vi "handleMode.vi"(8 "error in (no error)":errorcluster, 10 "stepName":T1, 11 "Stand in":refnum<class "Stand.lvclass">) -> (0 "error out":errorcluster, 3 "Stand out":refnum<class "Stand.lvclass">)   [LabVIEW 2019, in "Stand.lvclass"]
uses:
  Stand.lvclass
  FPGA/TypeDef/DO index.ctl
  Valve_2DO_2DI_class/Valve_2DO_2DI.lvclass
  TypeDef/Direction.ctl
  Device_class/Device.lvclass
  FPGA_API_class/FPGA API.lvclass
  f638fa31-f737-482a-bde8-81f5a2056bae.vi
  PM_Group_class/PM_Group.lvclass
  TypeDef/Motor N.ctl
  TypeDef/Active Motor.ctl
  MessageInterface_class/MessageInterface.lvclass
  TypeDef/Step_Name.ctl
  FPGA/TypeDef/AI index.ctl
  AI_class/AI.lvclass
  NeedleValve_class/NeedleValve.lvclass
  D:/GIT H4000/H4000/src/Device_class/Device.lvclass
  D:/GIT H4000/H4000/src/Proccess_class/Proccess.lvclass
  ExpFitter/ExpFitter.lvclass
  TypeDef/Needle Valve State.ctl
  LinealFitting/LinealFitting.lvclass
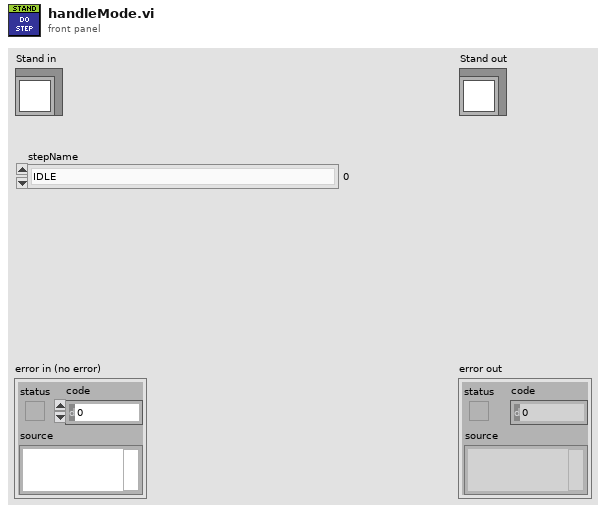
[diagram p1: front panel]
types:
  T1 = typedef "Step_Name.ctl" = enum16{"IDLE", "Filling", "Low Pressure", "Hi Pressure", "Abrupt Pressure Release", "Smooth Pressure Release", "Measuring Leakage Sensor 41.3", "Measuring Leakage Burette 42", "Alarm", "Stop Pump"}
  T2 = typedef "Direction.ctl" = enum16{"None", "DUT", "Chamber"}
  T3 = typedef "Active Motor.ctl" = cluster{"Active":bool, "MotorN":T4}
  T4 = typedef "Motor N.ctl" = enum16{"M12", "M21", "M24"}
  T5 = typedef "Step_Name.ctl" = enum16{"NONE", "Filling DUT", "Filling Chamber", "Pressure Up DUT", "Abrupt Pressure Release DUT", "Smooth Pressure Release DUT", "Pressure Up Chamber", "Abrupt Pressure Release Chamber", "Smooth Pressure Release Chamber", "Measuring leakage sensor 41.3", "Measuring leakage burette 42", "Low Pressure DUT", "Low Pressure Chamber", "Low Pressure HPP", "ALARM", "Open Air", "MicroStep DUT", "MicroStep CMBR", "Stop Pump", "Press Down by Valve DUT"}
  T6 = typedef "Needle Valve State.ctl" = enum16{"STOPED", "CLOSED", "OPENED", "OPENING", "CLOSING"}
  T7 = typedef "DO index.ctl" = u8
  T8 = typedef "AI index.ctl" = u8
  T9 = typedef "AI_Data.ctl" = cluster{"Stat Data":T10, "OutOfRangeMax":bool, "OutOfRangeMin":bool, "HIHI":bool, "HI":bool, "LO":bool, "LOLO":bool, "DATA N":T11, "DATA PERIOD":T11, "UPPER TH":dbl, "LOWER TH":dbl}
  T10 = typedef "AI Statistics Data.ctl" = cluster{"raw mean":dbl, "scl mean":dbl, "raw mean 1Hz":dbl, "scl mean 1Hz":dbl}
  T11 = typedef "DATA Oscill.ctl" = cluster{"SUM":dbl, "COUNTER":dbl, "MAX CURR":dbl, "MIN CURR":dbl, "AVR":dbl, "MAX":dbl, "MIN":dbl, "DELTA AVR":dbl, "DELTA MAX":dbl, "DELTA MIN":dbl, "PERIOD":dbl}
  T12 = typedef "Needle Valve Data.ctl" = cluster{"Engine State":T13, "StateValveModbus":T6, "Alarms":T14, "RAW":i32, "Angele":dbl, "Step":i32, "Encoder":i32, "Kinematic":T15, "Limits":T16, "EncoderMax":i32, "Counter Max Dont Update":i32, "EncoderMin":i32, "Counter Min Dont Update":i32, "Prepere Counter":i32, "STEP INIT":i32, "offset - Angel":dbl}
  T13 = typedef "MB_ENGINE.lvclass/Engine State.ctl" = u16
  T14 = typedef "MB_ENGINE.lvclass/Engine Alarms.ctl" = cluster{"OL":bool, "TF":bool, "STL":bool, "OCP":bool, "CPUV":bool, "UVLO":bool, "SPI_ERROR":bool, "Fault":bool, "OL 2":bool, "TF 2":bool, "STL 2":bool, "OCP 2":bool, "CPUV 2":bool, "UVLO 2":bool, "reserved":bool, "InitDone":bool}
  T15 = typedef "MB_ENGINE.lvclass/Settings.ctl" = cluster{"ACC Steps Per Sec^2":u16, "DEC Steps Per Sec^2":u16, "Min Velosity Step Per Sec":u16, "Max Velosity Step Per Sec":u16, "MicroStep":u16}
  T16 = typedef "MB_ENGINE.lvclass/Limits Status.ctl" = cluster{"Fault 2 Switch":bool, "Fault 1 Switch":bool, "Center(Home)":bool, "Lower Limit":bool, "Upper Limit":bool}
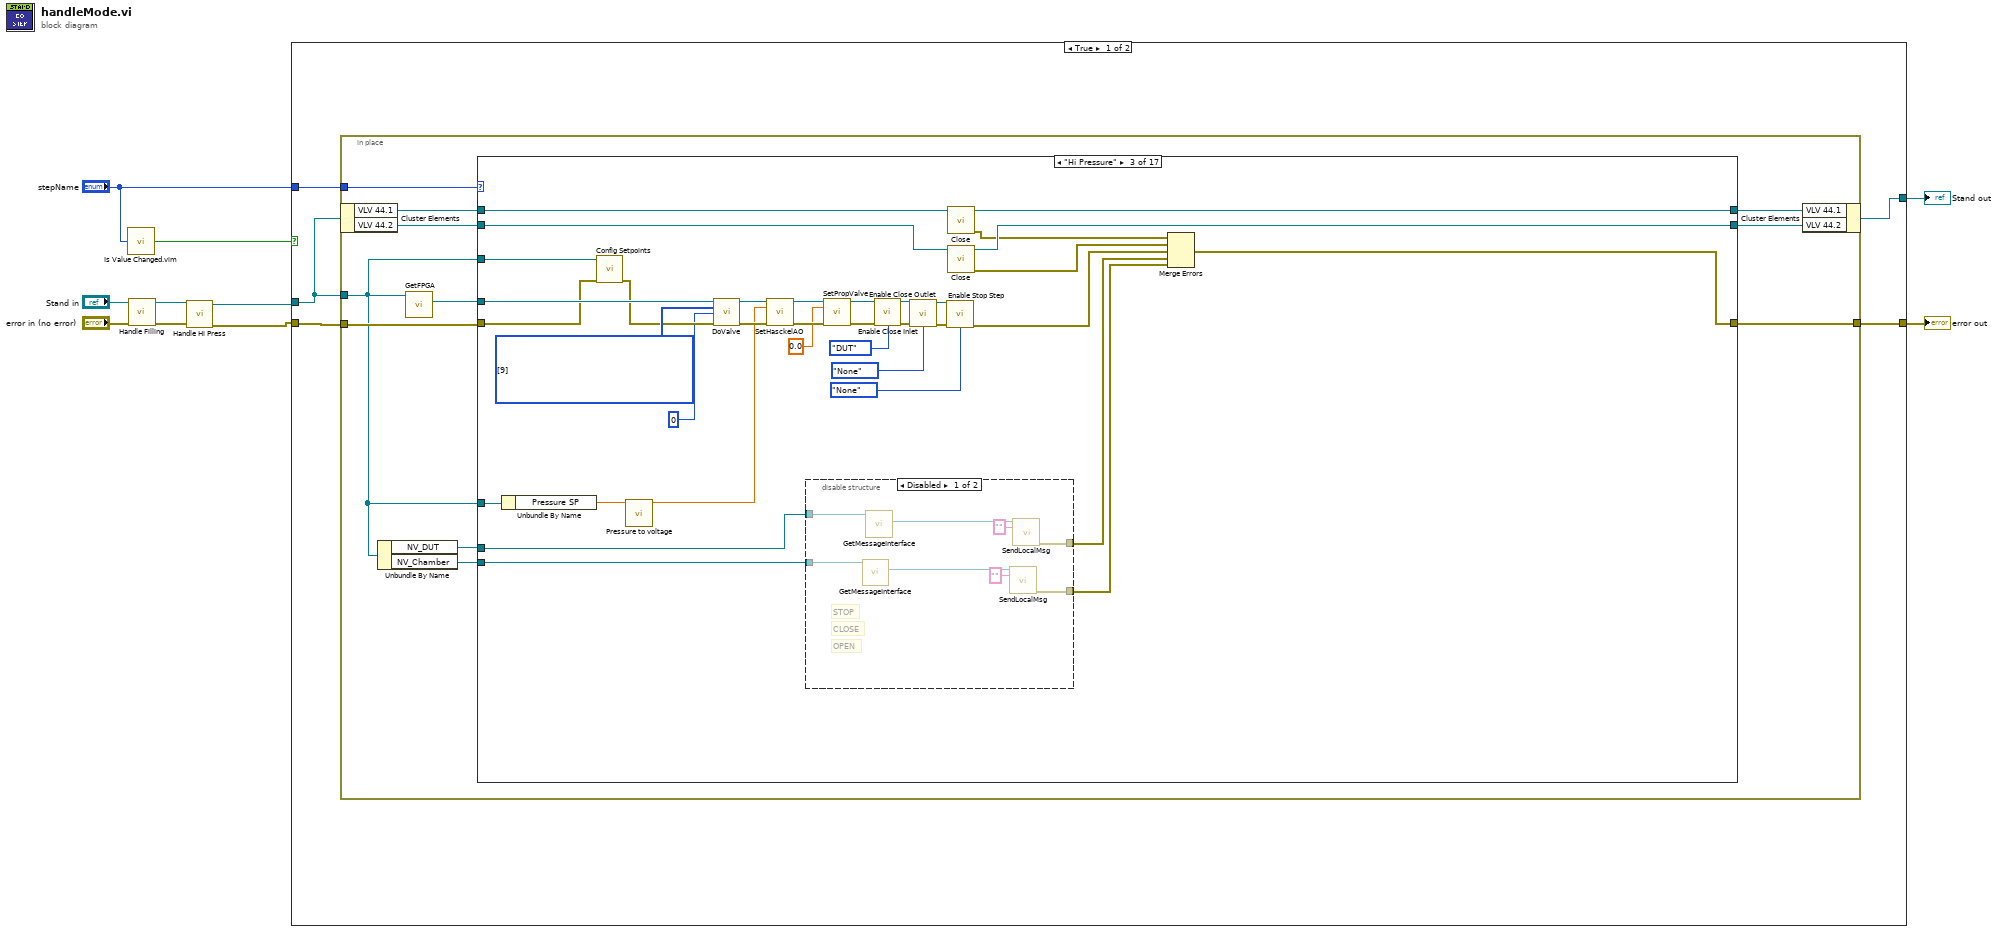
[diagram p0: block diagram]
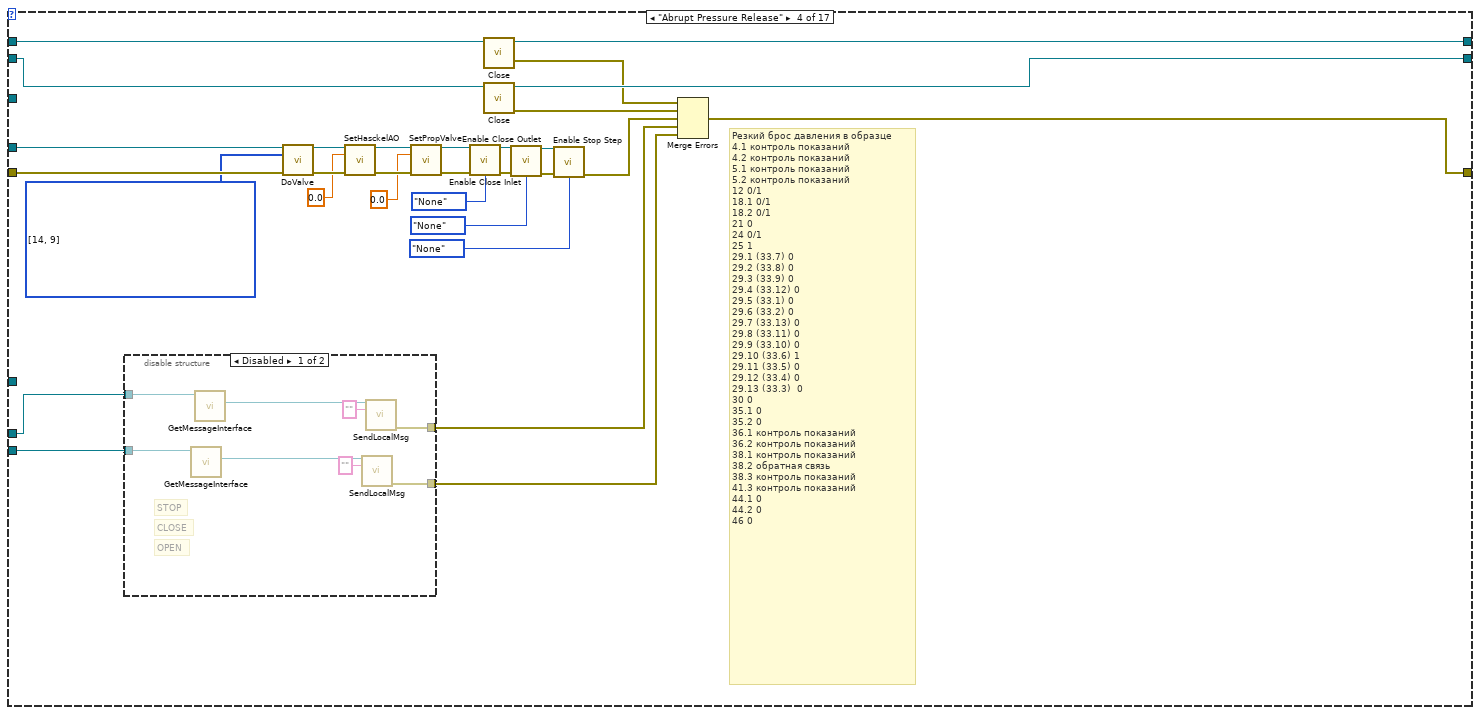
[diagram p5: hidden frame]
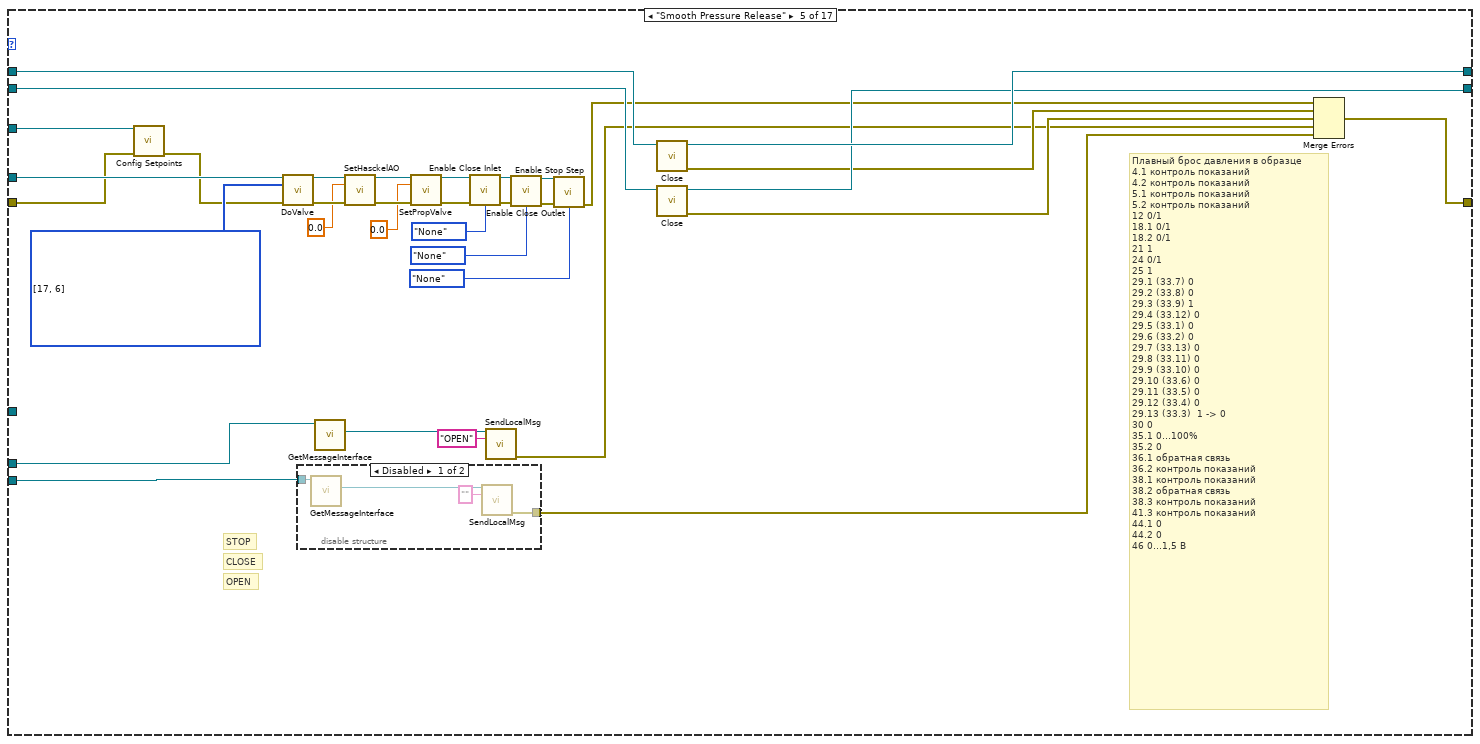
[diagram p7: hidden frame]
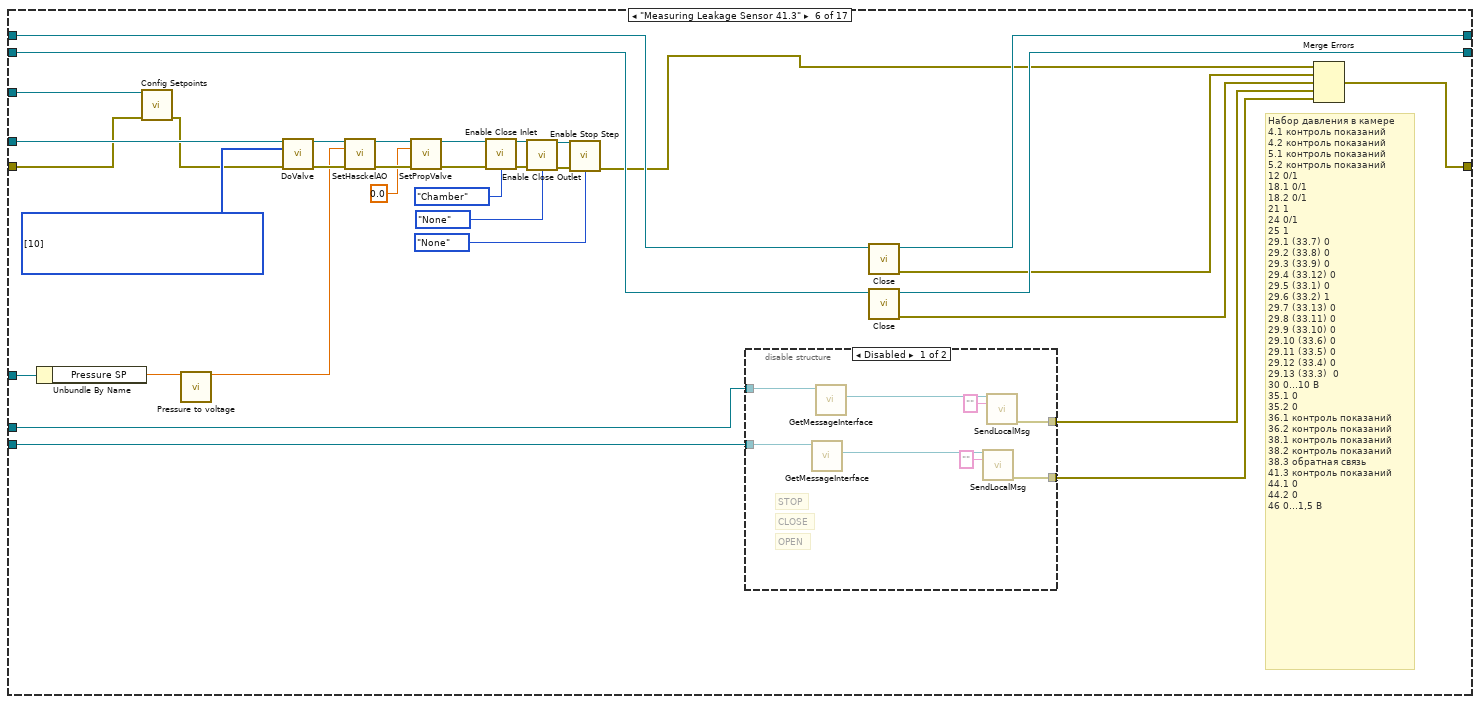
[diagram p9: hidden frame]
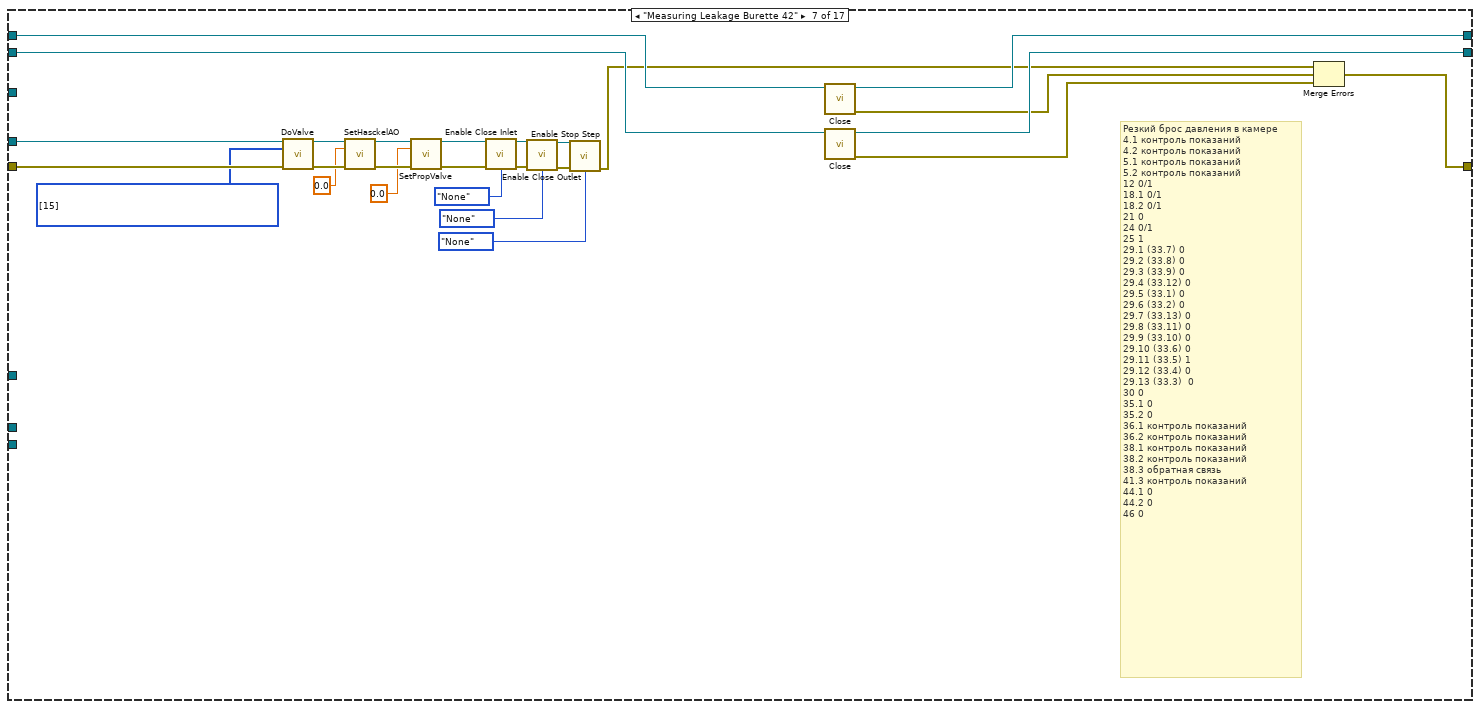
[diagram p11: hidden frame]
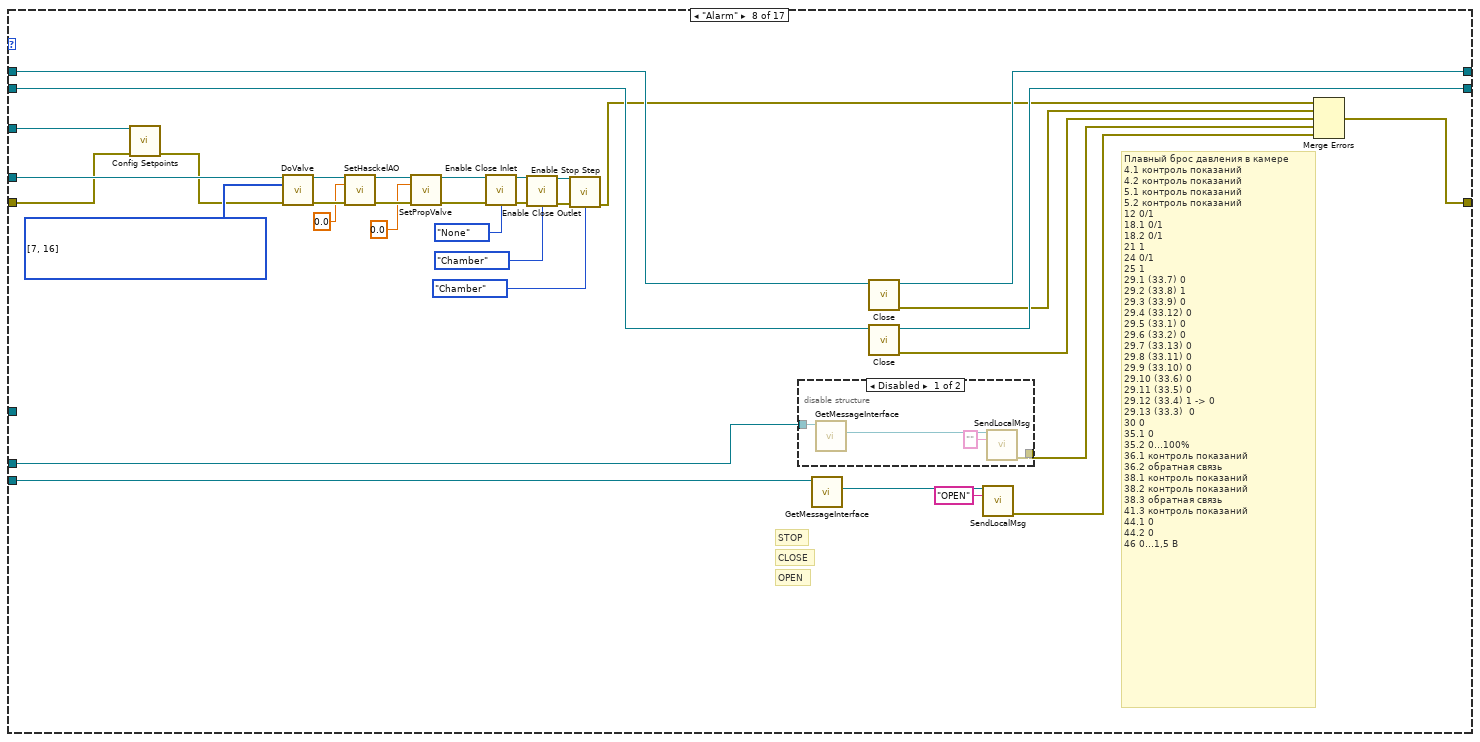
[diagram p12: hidden frame]
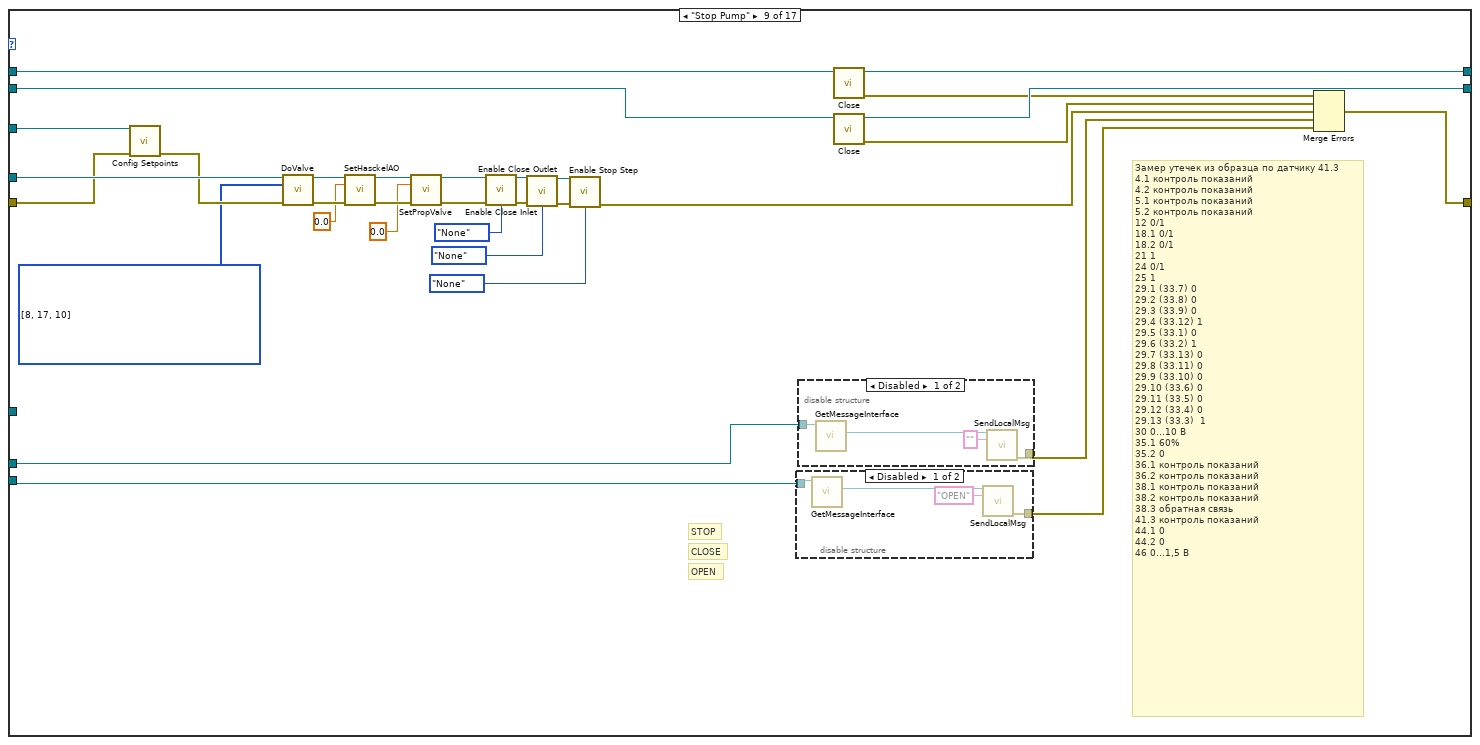
[diagram p14: hidden frame]
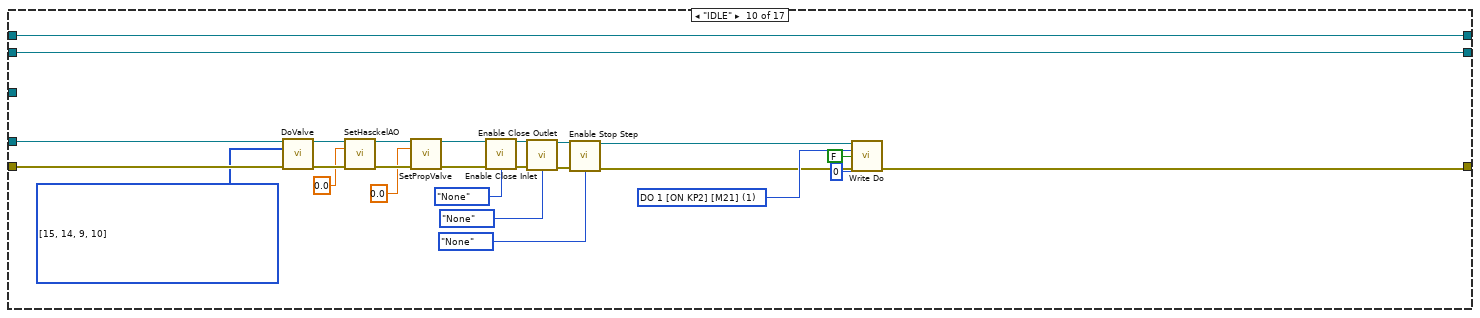
[diagram p17: hidden frame]
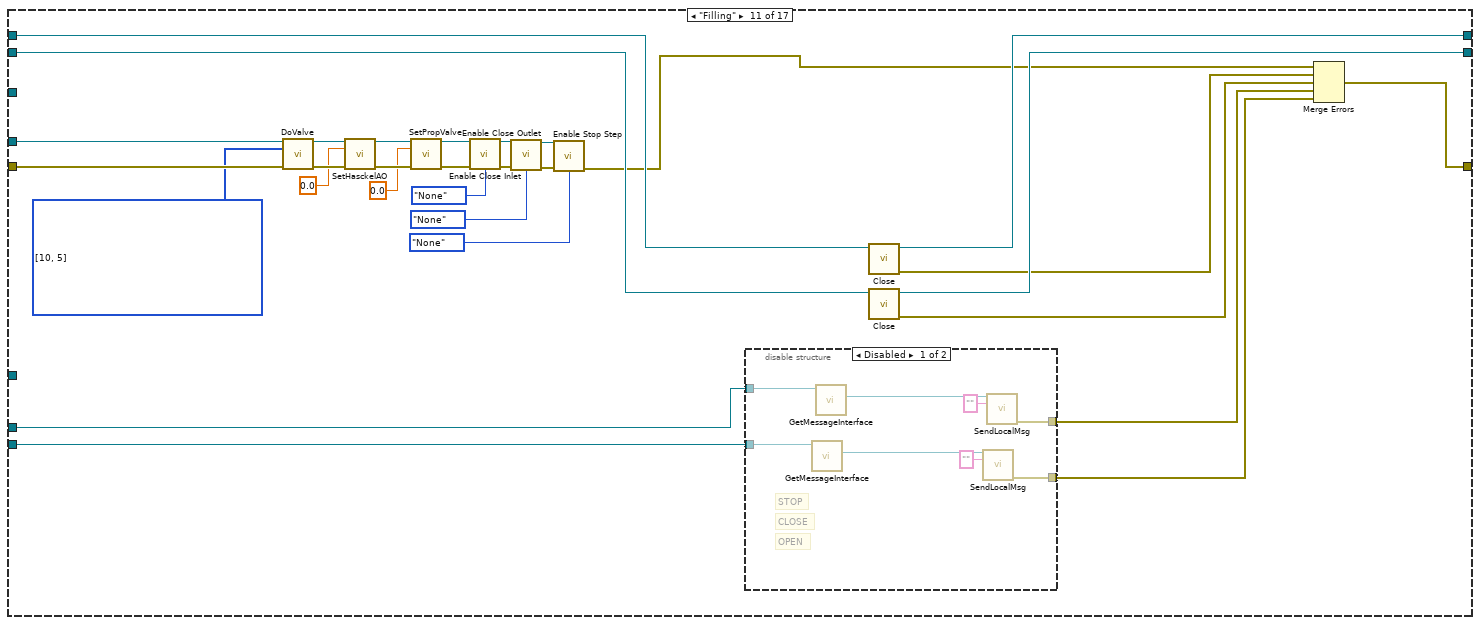
[diagram p18: hidden frame]
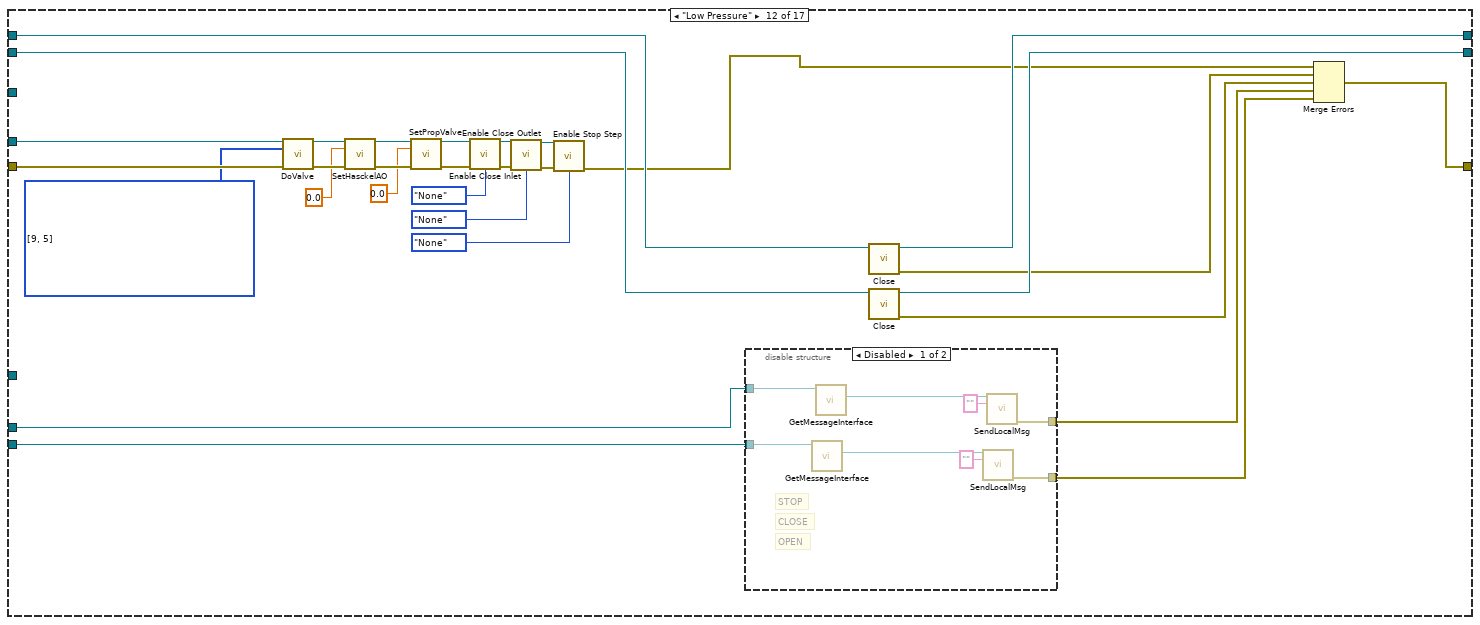
[diagram p20: hidden frame]
diagram:
  n1 = call "Is Value Changed.vim"("value"="stepName") -> ("changed or first call?"=w9:bool)
  n2 = call "Handle Filling.vi"("error in (no error)"="error in (no error)", "Stand in"="Stand in") -> ("error out"=w3:errorcluster, "Stand out"=w4:refnum<class "Stand.lvclass">)  [unwired: 8 in]
  n3 = call "Handle Hi Press.vi"("error in (no error)"=w3, "Stand in"=w4) -> ("error out"=w1:errorcluster, "Stand out"=w2:refnum<class "Stand.lvclass">)  [unwired: 8 in]
  n4 = case shown="True" w9 {
    tunnel: "stepName" -> [w15 _]
    tunnel: w2 -> [w13 w583]
    tunnel: w1 -> [w14 w584]
    tunnel: [w12 w582] -> w8
    tunnel: [w11 w581] -> w7
    frame True {
      n5 = in-place {
        in-place-border: w15 -> [w26]
        in-place-border: [w25] -> w11
        in-place-border: w14 -> [w24]
        in-place-border: w13 -> [w16]
        n6 = in-place-cluster #1(w13) -> ("VLV 44.1"=w22:refnum<class "Valve_2DO_2DI.lvclass">, "VLV 44.2"=w21:refnum<class "Valve_2DO_2DI.lvclass">)
        n7 = Unbundle By Name(w16) -> ("NV_DUT"=w18:refnum<class "NeedleValve.lvclass">, "NV_Chamber"=w17:refnum<class "NeedleValve.lvclass">)
        n8 = call "GetFPGA.vi"("Device in"=w16) -> ("FPGA API.lvclass"=w23:refnum<class "FPGA API.lvclass">)  [unwired: 10 in]
        n9 = case shown="\"Hi Pressure\"" w26 {
          tunnel: w24 -> [w29 _ w35 w102 w114 w150 w216 w218 w258 w320 w350 w388 w426 w437 w489 w523 w549]
          tunnel: [w29 _ w54 w92 w135 w172 w206 w241 w277 w296 w340 w378 w416 w458 w495 w529 w568] -> w25
          tunnel: w22 -> [w28 _ w59 w96 w139 w177 w210 w245 w281 w314 w344 w382 w420 w463 w505 w539 w570]
          tunnel: w21 -> [w27 _ w56 w94 w137 w174 w208 w243 w279 w313 w342 w380 w418 w460 w504 w538 w569]
          tunnel: w23 -> [_ _ w60 w97 w140 w178 w211 w246 w282 w315 w345 w383 w421 w464 w506 w540 w550]
          tunnel: w16 -> [_ _ w58 _ _ w176 _ _ _ _ _ _ _ w462 w482 w516 _]
          tunnel: [w28 _ w57 w95 w138 w175 w209 w244 w280 w314 w343 w381 w419 w461 w505 w539 w570] -> w20
          tunnel: [w27 _ w55 w93 w136 w173 w207 w242 w278 w313 w341 w379 w417 w459 w504 w538 w569] -> w19
          tunnel: w18 -> [_ _ w53 w91 w132 w169 _ w238 w274 _ w337 w375 w413 w455 _ _ w567]
          tunnel: w17 -> [_ _ w51 w89 w130 w167 _ w236 w272 _ w335 w373 w411 w453 _ _ w565]
          tunnel: w16 -> [_ _ w36 _ w115 w151 _ w219 w259 _ _ _ _ w438 w490 w524 _]
          frame "IDLE" {
          }
          frame "Low Pressure" {
          }
          frame "Hi Pressure" {
            w40 = T7[] [9] items=["DO 0 [KP1] [M12]", "DO 1 [ON KP2] [M21]", "DO 2 [ON KP3] [M24]", "DO 3 [WATER Y18.1 [DO3]]", "DO 4 [WATER Y18.2 [DO4]]", "DO 5 [KP6 Y29.1 33.7]", "DO 6 [KP7 Y29.2 33.8]", "DO 7 [KP8 Y29.3 33.9]", "DO 8 [KP9 Y29.4  33.12]", "DO 9 [KP10 Y29.5 33.1]", "DO 10 [KP11 Y29.6 33.2]", "DO 11 [KP12 Y29.7  33.13]", "DO 12 [KP13 Y29.8  33.11]", "DO 13 [KP14 Y29.9 33.10]", "DO 14 [KP15 Y29.10  33.6]", "DO 15 [KP16 Y29.11  33.5]", "DO 16 [KP17 Y29.12  33.4]", "DO 17 [KP18 Y29.13 33.3]", "DO 18 [AIR KP19]", "DO 19 [STEP DRIVE EN KP20]", "DO 20 [KP21 Y44.1 OPEN]", "DO 21 [ KP22 Y44.1 CLOSE]", "DO 22 [ KP23 Y44.2 OPEN]", "DO 23", "DO 24 [STEP DRIVE 1]", "DO 25 [STEP DRIVE 2]"] ("#DO")
            n10 = Unbundle By Name(w58) -> ("Pressure SP"=w38:dbl)
            n11 = call "Config Setpoints.vi"("reference in"=w36, "error in (no error)"=w35) -> ("error out"=w34:errorcluster)  [unwired: 13 in]
            n12 = call "Pressure to voltage.vi"("Pressure SP"=w38) -> ("Voltage"=w37:dbl)  [unwired: 14 in]
            n13 = call "DoValve.vi"("reference in"=w60, 5:w40, 7:u32 0 ("Time uSec"), "error in (no error)"=w34) -> ("reference out"=w64:refnum<class "FPGA API.lvclass">, "error out"=w63:errorcluster)  [unwired: 10 in]
            n14 = call-dynamic "SetHasckelAO.vi"("FPGA API in"=w64, "Haskel in"=w37, "error in (no error)"=w63) -> ("FPGA API out"=w62:refnum<class "FPGA API.lvclass">, "error out"=w61:errorcluster)  [unwired: 11 in]
            n15 = disable-structure shown="Disabled" {
              disable-tunnel: w53 -> [w72 _]
              disable-tunnel: [w70 _] -> w52
              disable-tunnel: w51 -> [w68 _]
              disable-tunnel: [w65 _] -> w41
              frame Disabled {
                # "OPEN"
                # "CLOSE"
                # "STOP"
                n16 = call "GetMessageInterface.vi"("Device in"=w68) -> ("MessageInterface"=w69:refnum<class "MessageInterface.lvclass">)  [unwired: 10 in]
                n17 = call "GetMessageInterface.vi"("Device in"=w72) -> ("MessageInterface"=w71:refnum<class "MessageInterface.lvclass">)  [unwired: 10 in]
                n18 = call-dynamic "SendLocalMsg.vi"("reference in"=w69, "name"="") -> ("error out"=w65:errorcluster)  [unwired: 11 in, 2 out]
                n19 = call-dynamic "SendLocalMsg.vi"("reference in"=w71, "name"="") -> ("error out"=w70:errorcluster)  [unwired: 11 in, 2 out]
              }
              frame Enabled {
              }
            }
            n20 = call-dynamic "SetPropValve.vi"("FPGA API in"=w62, "AO 1"=0.0, "error in (no error)"=w61) -> ("FPGA API out"=w50:refnum<class "FPGA API.lvclass">, "error out"=w49:errorcluster)  [unwired: 11 in]
            n21 = call-dynamic "Enable Close Inlet.vi"("FPGA API in"=w50, "error in (no error)"=w49, "Direction"=Direction."DUT") -> ("FPGA API out"=w47:refnum<class "FPGA API.lvclass">, "error out"=w46:errorcluster)  [unwired: 11 in]
            n22 = call-dynamic "Enable Close Outlet.vi"("FPGA API in"=w47, "error in (no error)"=w46, "Direction"=Direction."None") -> ("FPGA API out"=w44:refnum<class "FPGA API.lvclass">, "error out"=w43:errorcluster)  [unwired: 11 in]
            n23 = call-dynamic "Enable Stop Step.vi"("FPGA API in"=w44, "error in (no error)"=w43, "Direction"=Direction."None") -> ("error out"=w33:errorcluster)  [unwired: 11 in, 1 out]
            n24 = call "Close.vi"("Pump_1AI_1DO_2DI in"=w59) -> ("error out"=w31:errorcluster, "Pump_1AI_1DO_2DI out"=w57:refnum<class "Valve_2DO_2DI.lvclass">)  [unwired: 9 in]
            n25 = call "Close.vi"("Pump_1AI_1DO_2DI in"=w56) -> ("error out"=w32:errorcluster, "Pump_1AI_1DO_2DI out"=w55:refnum<class "Valve_2DO_2DI.lvclass">)  [unwired: 9 in]
            n26 = Merge Errors(w31, w32, w33, w52, w41) -> (w54:errorcluster)
          }
          frame "Abrupt Pressure Release" {
            w77 = T7[] [14, 9] items=["DO 0 [KP1] [M12]", "DO 1 [ON KP2] [M21]", "DO 2 [ON KP3] [M24]", "DO 3 [WATER Y18.1 [DO3]]", "DO 4 [WATER Y18.2 [DO4]]", "DO 5 [KP6 Y29.1 33.7]", "DO 6 [KP7 Y29.2 33.8]", "DO 7 [KP8 Y29.3 33.9]", "DO 8 [KP9 Y29.4  33.12]", "DO 9 [KP10 Y29.5 33.1]", "DO 10 [KP11 Y29.6 33.2]", "DO 11 [KP12 Y29.7  33.13]", "DO 12 [KP13 Y29.8  33.11]", "DO 13 [KP14 Y29.9 33.10]", "DO 14 [KP15 Y29.10  33.6]", "DO 15 [KP16 Y29.11  33.5]", "DO 16 [KP17 Y29.12  33.4]", "DO 17 [KP18 Y29.13 33.3]", "DO 18 [AIR KP19]", "DO 19 [STEP DRIVE EN KP20]", "DO 20 [KP21 Y44.1 OPEN]", "DO 21 [ KP22 Y44.1 CLOSE]", "DO 22 [ KP23 Y44.2 OPEN]", "DO 23", "DO 24 [STEP DRIVE 1]", "DO 25 [STEP DRIVE 2]"] ("#DO")
            # "Резкий брос давления в образце\n4.1\tконтроль показаний\n4.2\tконтроль показаний\n5.1\tконтроль показаний\n5.2\tконтроль показаний\n12\t0/1\n18.1\t0/1\n18.2\t0/1\n21\t0\n24\t0/1\n25\t1\n29.1 (33.7)\t0\n29.2 (33.8)\t0\n29.3 (33.9)\t0\n29.4 (33.12)\t0\n29.5 (33.1)\t0\n29.6 (33.2)\t0\n29.7 (33.13)\t0\n29.8 (33.11)\t0\n29.9 (33.10)\t0\n29.10 (33.6)\t1\n29.11 (33.5)\t0\n29.12 (33.4)\t0\n29.13 (33.3) \t0\n30\t0\n35.1\t0\n35.2\t0\n36.1\tконтроль показаний\n36.2\tконтроль показаний\n38.1\tконтроль показаний\n38.2\tобратная связь\n38.3\tконтроль показаний\n41.3\tконтроль показаний\n44.1\t0\n44.2\t0\n46\t0"
            n27 = disable-structure shown="Disabled" {
              disable-tunnel: w91 -> [w110 _]
              disable-tunnel: [w108 _] -> w90
              disable-tunnel: w89 -> [w106 _]
              disable-tunnel: [w103 _] -> w79
              frame Disabled {
                # "OPEN"
                # "CLOSE"
                # "STOP"
                n28 = call "GetMessageInterface.vi"("Device in"=w106) -> ("MessageInterface"=w107:refnum<class "MessageInterface.lvclass">)  [unwired: 10 in]
                n29 = call "GetMessageInterface.vi"("Device in"=w110) -> ("MessageInterface"=w109:refnum<class "MessageInterface.lvclass">)  [unwired: 10 in]
                n30 = call-dynamic "SendLocalMsg.vi"("reference in"=w107, "name"="") -> ("error out"=w103:errorcluster)  [unwired: 11 in, 2 out]
                n31 = call-dynamic "SendLocalMsg.vi"("reference in"=w109, "name"="") -> ("error out"=w108:errorcluster)  [unwired: 11 in, 2 out]
              }
              frame Enabled {
              }
            }
            n32 = call "DoValve.vi"("reference in"=w97, 5:w77, "error in (no error)"=w102) -> ("reference out"=w101:refnum<class "FPGA API.lvclass">, "error out"=w100:errorcluster)  [unwired: 11 in]
            n33 = call-dynamic "SetHasckelAO.vi"("FPGA API in"=w101, "Haskel in"=0.0, "error in (no error)"=w100) -> ("FPGA API out"=w99:refnum<class "FPGA API.lvclass">, "error out"=w98:errorcluster)  [unwired: 11 in]
            n34 = call-dynamic "SetPropValve.vi"("FPGA API in"=w99, "AO 1"=0.0, "error in (no error)"=w98) -> ("FPGA API out"=w88:refnum<class "FPGA API.lvclass">, "error out"=w87:errorcluster)  [unwired: 11 in]
            n35 = call-dynamic "Enable Close Inlet.vi"("FPGA API in"=w88, "error in (no error)"=w87, "Direction"=Direction."None") -> ("FPGA API out"=w85:refnum<class "FPGA API.lvclass">, "error out"=w84:errorcluster)  [unwired: 11 in]
            n36 = call "Close.vi"("Pump_1AI_1DO_2DI in"=w96) -> ("error out"=w74:errorcluster, "Pump_1AI_1DO_2DI out"=w95:refnum<class "Valve_2DO_2DI.lvclass">)  [unwired: 9 in]
            n37 = call "Close.vi"("Pump_1AI_1DO_2DI in"=w94) -> ("error out"=w75:errorcluster, "Pump_1AI_1DO_2DI out"=w93:refnum<class "Valve_2DO_2DI.lvclass">)  [unwired: 9 in]
            n38 = call-dynamic "Enable Close Outlet.vi"("FPGA API in"=w85, "error in (no error)"=w84, "Direction"=Direction."None") -> ("FPGA API out"=w82:refnum<class "FPGA API.lvclass">, "error out"=w81:errorcluster)  [unwired: 11 in]
            n39 = call-dynamic "Enable Stop Step.vi"("FPGA API in"=w82, "error in (no error)"=w81, "Direction"=Direction."None") -> ("error out"=w73:errorcluster)  [unwired: 11 in, 1 out]
            n40 = Merge Errors(w74, w75, w73, w90, w79) -> (w92:errorcluster)
          }
          frame "Smooth Pressure Release" {
            w117 = T7[] [17, 6] items=["DO 0 [KP1] [M12]", "DO 1 [ON KP2] [M21]", "DO 2 [ON KP3] [M24]", "DO 3 [WATER Y18.1 [DO3]]", "DO 4 [WATER Y18.2 [DO4]]", "DO 5 [KP6 Y29.1 33.7]", "DO 6 [KP7 Y29.2 33.8]", "DO 7 [KP8 Y29.3 33.9]", "DO 8 [KP9 Y29.4  33.12]", "DO 9 [KP10 Y29.5 33.1]", "DO 10 [KP11 Y29.6 33.2]", "DO 11 [KP12 Y29.7  33.13]", "DO 12 [KP13 Y29.8  33.11]", "DO 13 [KP14 Y29.9 33.10]", "DO 14 [KP15 Y29.10  33.6]", "DO 15 [KP16 Y29.11  33.5]", "DO 16 [KP17 Y29.12  33.4]", "DO 17 [KP18 Y29.13 33.3]", "DO 18 [AIR KP19]", "DO 19 [STEP DRIVE EN KP20]", "DO 20 [KP21 Y44.1 OPEN]", "DO 21 [ KP22 Y44.1 CLOSE]", "DO 22 [ KP23 Y44.2 OPEN]", "DO 23", "DO 24 [STEP DRIVE 1]", "DO 25 [STEP DRIVE 2]"] ("#DO")
            # "OPEN"
            # "CLOSE"
            # "STOP"
            # "Плавный брос давления в образце\n4.1\tконтроль показаний\n4.2\tконтроль показаний\n5.1\tконтроль показаний\n5.2\tконтроль показаний\n12\t0/1\n18.1\t0/1\n18.2\t0/1\n21\t1\n24\t0/1\n25\t1\n29.1 (33.7)\t0\n29.2 (33.8)\t0\n29.3 (33.9)\t1\n29.4 (33.12)\t0\n29.5 (33.1)\t0\n29.6 (33.2)\t0\n29.7 (33.13)\t0\n29.8 (33.11)\t0\n29.9 (33.10)\t0\n29.10 (33.6)\t0\n29.11 (33.5)\t0\n29.12 (33.4)\t0\n29.13 (33.3) \t1 -> 0\n30\t0\n35.1\t0…100%\n35.2\t0\n36.1\tобратная связь\n36.2\tконтроль показаний\n38.1\tконтроль показаний\n38.2\tобратная связь\n38.3\tконтроль показаний\n41.3\tконтроль показаний\n44.1\t0\n44.2\t0\n46\t0…1,5 В"
            n41 = call "Config Setpoints.vi"("reference in"=w115, "error in (no error)"=w114) -> ("error out"=w113:errorcluster)  [unwired: 13 in]
            n42 = call "DoValve.vi"("reference in"=w140, 5:w117, "error in (no error)"=w113) -> ("reference out"=w144:refnum<class "FPGA API.lvclass">, "error out"=w143:errorcluster)  [unwired: 11 in]
            n43 = disable-structure shown="Disabled" {
              disable-tunnel: w130 -> [w148 _]
              disable-tunnel: [w147 _] -> w119
              frame Disabled {
                n44 = call "GetMessageInterface.vi"("Device in"=w148) -> ("MessageInterface"=w146:refnum<class "MessageInterface.lvclass">)  [unwired: 10 in]
                n45 = call-dynamic "SendLocalMsg.vi"("reference in"=w146, "name"="") -> ("error out"=w147:errorcluster)  [unwired: 11 in, 2 out]
              }
              frame Enabled {
              }
            }
            n46 = call "GetMessageInterface.vi"("Device in"=w132) -> ("MessageInterface"=w112:refnum<class "MessageInterface.lvclass">)  [unwired: 10 in]
            n47 = call-dynamic "SetHasckelAO.vi"("FPGA API in"=w144, "Haskel in"=0.0, "error in (no error)"=w143) -> ("FPGA API out"=w142:refnum<class "FPGA API.lvclass">, "error out"=w141:errorcluster)  [unwired: 11 in]
            n48 = call-dynamic "SetPropValve.vi"("FPGA API in"=w142, "AO 1"=0.0, "error in (no error)"=w141) -> ("FPGA API out"=w129:refnum<class "FPGA API.lvclass">, "error out"=w128:errorcluster)  [unwired: 11 in]
            n49 = call-dynamic "Enable Close Inlet.vi"("FPGA API in"=w129, "error in (no error)"=w128, "Direction"=Direction."None") -> ("FPGA API out"=w126:refnum<class "FPGA API.lvclass">, "error out"=w125:errorcluster)  [unwired: 11 in]
            n50 = call-dynamic "SendLocalMsg.vi"("reference in"=w112, "name"="OPEN") -> ("error out"=w131:errorcluster)  [unwired: 11 in, 2 out]
            n51 = call-dynamic "Enable Close Outlet.vi"("FPGA API in"=w126, "error in (no error)"=w125, "Direction"=Direction."None") -> ("FPGA API out"=w123:refnum<class "FPGA API.lvclass">, "error out"=w122:errorcluster)  [unwired: 11 in]
            n52 = call-dynamic "Enable Stop Step.vi"("FPGA API in"=w123, "error in (no error)"=w122, "Direction"=Direction."None") -> ("error out"=w121:errorcluster)  [unwired: 11 in, 1 out]
            n53 = call "Close.vi"("Pump_1AI_1DO_2DI in"=w139) -> ("error out"=w133:errorcluster, "Pump_1AI_1DO_2DI out"=w138:refnum<class "Valve_2DO_2DI.lvclass">)  [unwired: 9 in]
            n54 = call "Close.vi"("Pump_1AI_1DO_2DI in"=w137) -> ("error out"=w134:errorcluster, "Pump_1AI_1DO_2DI out"=w136:refnum<class "Valve_2DO_2DI.lvclass">)  [unwired: 9 in]
            n55 = Merge Errors(w121, w133, w134, w131, w119) -> (w135:errorcluster)
          }
          frame "Measuring Leakage Sensor 41.3" {
            w152 = T7[] [10] items=["DO 0 [KP1] [M12]", "DO 1 [ON KP2] [M21]", "DO 2 [ON KP3] [M24]", "DO 3 [WATER Y18.1 [DO3]]", "DO 4 [WATER Y18.2 [DO4]]", "DO 5 [KP6 Y29.1 33.7]", "DO 6 [KP7 Y29.2 33.8]", "DO 7 [KP8 Y29.3 33.9]", "DO 8 [KP9 Y29.4  33.12]", "DO 9 [KP10 Y29.5 33.1]", "DO 10 [KP11 Y29.6 33.2]", "DO 11 [KP12 Y29.7  33.13]", "DO 12 [KP13 Y29.8  33.11]", "DO 13 [KP14 Y29.9 33.10]", "DO 14 [KP15 Y29.10  33.6]", "DO 15 [KP16 Y29.11  33.5]", "DO 16 [KP17 Y29.12  33.4]", "DO 17 [KP18 Y29.13 33.3]", "DO 18 [AIR KP19]", "DO 19 [STEP DRIVE EN KP20]", "DO 20 [KP21 Y44.1 OPEN]", "DO 21 [ KP22 Y44.1 CLOSE]", "DO 22 [ KP23 Y44.2 OPEN]", "DO 23", "DO 24 [STEP DRIVE 1]", "DO 25 [STEP DRIVE 2]"] ("#DO")
            # "Набор давления в камере\n4.1\tконтроль показаний\n4.2\tконтроль показаний\n5.1\tконтроль показаний\n5.2\tконтроль показаний\n12\t0/1\n18.1\t0/1\n18.2\t0/1\n21\t1\n24\t0/1\n25\t1\n29.1 (33.7)\t0\n29.2 (33.8)\t0\n29.3 (33.9)\t0\n29.4 (33.12)\t0\n29.5 (33.1)\t0\n29.6 (33.2)\t1\n29.7 (33.13)\t0\n29.8 (33.11)\t0\n29.9 (33.10)\t0\n29.10 (33.6)\t0\n29.11 (33.5)\t0\n29.12 (33.4)\t0\n29.13 (33.3) \t0\n30\t0…10 В\n35.1\t0\n35.2\t0\n36.1\tконтроль показаний\n36.2\tконтроль показаний\n38.1\tконтроль показаний\n38.2\tконтроль показаний\n38.3\tобратная связь\n41.3\tконтроль показаний\n44.1\t0\n44.2\t0\n46\t0…1,5 В"
            n56 = Unbundle By Name(w176) -> ("Pressure SP"=w154:dbl)
            n57 = call "Config Setpoints.vi"("reference in"=w151, "error in (no error)"=w150) -> ("error out"=w149:errorcluster)  [unwired: 13 in]
            n58 = call "Pressure to voltage.vi"("Pressure SP"=w154) -> ("Voltage"=w153:dbl)  [unwired: 14 in]
            n59 = call "DoValve.vi"("reference in"=w178, 5:w152, "error in (no error)"=w149) -> ("reference out"=w182:refnum<class "FPGA API.lvclass">, "error out"=w181:errorcluster)  [unwired: 11 in]
            n60 = call-dynamic "SetHasckelAO.vi"("FPGA API in"=w182, "Haskel in"=w153, "error in (no error)"=w181) -> ("FPGA API out"=w180:refnum<class "FPGA API.lvclass">, "error out"=w179:errorcluster)  [unwired: 11 in]
            n61 = call-dynamic "SetPropValve.vi"("FPGA API in"=w180, "AO 1"=0.0, "error in (no error)"=w179) -> ("FPGA API out"=w166:refnum<class "FPGA API.lvclass">, "error out"=w165:errorcluster)  [unwired: 11 in]
            n62 = call-dynamic "Enable Close Inlet.vi"("FPGA API in"=w166, "error in (no error)"=w165, "Direction"=Direction."Chamber") -> ("FPGA API out"=w163:refnum<class "FPGA API.lvclass">, "error out"=w162:errorcluster)  [unwired: 11 in]
            n63 = call-dynamic "Enable Close Outlet.vi"("FPGA API in"=w163, "error in (no error)"=w162, "Direction"=Direction."None") -> ("FPGA API out"=w160:refnum<class "FPGA API.lvclass">, "error out"=w159:errorcluster)  [unwired: 11 in]
            n64 = call-dynamic "Enable Stop Step.vi"("FPGA API in"=w160, "error in (no error)"=w159, "Direction"=Direction."None") -> ("error out"=w158:errorcluster)  [unwired: 11 in, 1 out]
            n65 = disable-structure shown="Disabled" {
              disable-tunnel: w169 -> [w190 _]
              disable-tunnel: [w188 _] -> w168
              disable-tunnel: w167 -> [w186 _]
              disable-tunnel: [w183 _] -> w156
              frame Disabled {
                # "OPEN"
                # "CLOSE"
                # "STOP"
                n66 = call "GetMessageInterface.vi"("Device in"=w186) -> ("MessageInterface"=w187:refnum<class "MessageInterface.lvclass">)  [unwired: 10 in]
                n67 = call "GetMessageInterface.vi"("Device in"=w190) -> ("MessageInterface"=w189:refnum<class "MessageInterface.lvclass">)  [unwired: 10 in]
                n68 = call-dynamic "SendLocalMsg.vi"("reference in"=w187, "name"="") -> ("error out"=w183:errorcluster)  [unwired: 11 in, 2 out]
                n69 = call-dynamic "SendLocalMsg.vi"("reference in"=w189, "name"="") -> ("error out"=w188:errorcluster)  [unwired: 11 in, 2 out]
              }
              frame Enabled {
              }
            }
            n70 = call "Close.vi"("Pump_1AI_1DO_2DI in"=w177) -> ("error out"=w170:errorcluster, "Pump_1AI_1DO_2DI out"=w175:refnum<class "Valve_2DO_2DI.lvclass">)  [unwired: 9 in]
            n71 = call "Close.vi"("Pump_1AI_1DO_2DI in"=w174) -> ("error out"=w171:errorcluster, "Pump_1AI_1DO_2DI out"=w173:refnum<class "Valve_2DO_2DI.lvclass">)  [unwired: 9 in]
            n72 = Merge Errors(w158, w170, w171, w168, w156) -> (w172:errorcluster)
          }
          frame "Measuring Leakage Burette 42" {
            w192 = T7[] [15] items=["DO 0 [KP1] [M12]", "DO 1 [ON KP2] [M21]", "DO 2 [ON KP3] [M24]", "DO 3 [WATER Y18.1 [DO3]]", "DO 4 [WATER Y18.2 [DO4]]", "DO 5 [KP6 Y29.1 33.7]", "DO 6 [KP7 Y29.2 33.8]", "DO 7 [KP8 Y29.3 33.9]", "DO 8 [KP9 Y29.4  33.12]", "DO 9 [KP10 Y29.5 33.1]", "DO 10 [KP11 Y29.6 33.2]", "DO 11 [KP12 Y29.7  33.13]", "DO 12 [KP13 Y29.8  33.11]", "DO 13 [KP14 Y29.9 33.10]", "DO 14 [KP15 Y29.10  33.6]", "DO 15 [KP16 Y29.11  33.5]", "DO 16 [KP17 Y29.12  33.4]", "DO 17 [KP18 Y29.13 33.3]", "DO 18 [AIR KP19]", "DO 19 [STEP DRIVE EN KP20]", "DO 20 [KP21 Y44.1 OPEN]", "DO 21 [ KP22 Y44.1 CLOSE]", "DO 22 [ KP23 Y44.2 OPEN]", "DO 23", "DO 24 [STEP DRIVE 1]", "DO 25 [STEP DRIVE 2]"] ("#DO")
            # "Резкий брос давления в камере\n4.1\tконтроль показаний\n4.2\tконтроль показаний\n5.1\tконтроль показаний\n5.2\tконтроль показаний\n12\t0/1\n18.1\t0/1\n18.2\t0/1\n21\t0\n24\t0/1\n25\t1\n29.1 (33.7)\t0\n29.2 (33.8)\t0\n29.3 (33.9)\t0\n29.4 (33.12)\t0\n29.5 (33.1)\t0\n29.6 (33.2)\t0\n29.7 (33.13)\t0\n29.8 (33.11)\t0\n29.9 (33.10)\t0\n29.10 (33.6)\t0\n29.11 (33.5)\t1\n29.12 (33.4)\t0\n29.13 (33.3) \t0\n30\t0\n35.1\t0\n35.2\t0\n36.1\tконтроль показаний\n36.2\tконтроль показаний\n38.1\tконтроль показаний\n38.2\tконтроль показаний\n38.3\tобратная связь\n41.3\tконтроль показаний\n44.1\t0\n44.2\t0\n46\t0"
            n73 = call "DoValve.vi"("reference in"=w211, 5:w192, "error in (no error)"=w216) -> ("reference out"=w215:refnum<class "FPGA API.lvclass">, "error out"=w214:errorcluster)  [unwired: 11 in]
            n74 = call-dynamic "SetHasckelAO.vi"("FPGA API in"=w215, "Haskel in"=0.0, "error in (no error)"=w214) -> ("FPGA API out"=w213:refnum<class "FPGA API.lvclass">, "error out"=w212:errorcluster)  [unwired: 11 in]
            n75 = call-dynamic "SetPropValve.vi"("FPGA API in"=w213, "AO 1"=0.0, "error in (no error)"=w212) -> ("FPGA API out"=w203:refnum<class "FPGA API.lvclass">, "error out"=w202:errorcluster)  [unwired: 11 in]
            n76 = call-dynamic "Enable Close Inlet.vi"("FPGA API in"=w203, "error in (no error)"=w202, "Direction"=Direction."None") -> ("FPGA API out"=w200:refnum<class "FPGA API.lvclass">, "error out"=w199:errorcluster)  [unwired: 11 in]
            n77 = call-dynamic "Enable Close Outlet.vi"("FPGA API in"=w200, "error in (no error)"=w199, "Direction"=Direction."None") -> ("FPGA API out"=w197:refnum<class "FPGA API.lvclass">, "error out"=w196:errorcluster)  [unwired: 11 in]
            n78 = call-dynamic "Enable Stop Step.vi"("FPGA API in"=w197, "error in (no error)"=w196, "Direction"=Direction."None") -> ("error out"=w195:errorcluster)  [unwired: 11 in, 1 out]
            n79 = call "Close.vi"("Pump_1AI_1DO_2DI in"=w210) -> ("error out"=w204:errorcluster, "Pump_1AI_1DO_2DI out"=w209:refnum<class "Valve_2DO_2DI.lvclass">)  [unwired: 9 in]
            n80 = call "Close.vi"("Pump_1AI_1DO_2DI in"=w208) -> ("error out"=w205:errorcluster, "Pump_1AI_1DO_2DI out"=w207:refnum<class "Valve_2DO_2DI.lvclass">)  [unwired: 9 in]
            n81 = Merge Errors(w195, w204, w205) -> (w206:errorcluster)
          }
          frame "Alarm" {
            w222 = T7[] [7, 16] items=["DO 0 [KP1] [M12]", "DO 1 [ON KP2] [M21]", "DO 2 [ON KP3] [M24]", "DO 3 [WATER Y18.1 [DO3]]", "DO 4 [WATER Y18.2 [DO4]]", "DO 5 [KP6 Y29.1 33.7]", "DO 6 [KP7 Y29.2 33.8]", "DO 7 [KP8 Y29.3 33.9]", "DO 8 [KP9 Y29.4  33.12]", "DO 9 [KP10 Y29.5 33.1]", "DO 10 [KP11 Y29.6 33.2]", "DO 11 [KP12 Y29.7  33.13]", "DO 12 [KP13 Y29.8  33.11]", "DO 13 [KP14 Y29.9 33.10]", "DO 14 [KP15 Y29.10  33.6]", "DO 15 [KP16 Y29.11  33.5]", "DO 16 [KP17 Y29.12  33.4]", "DO 17 [KP18 Y29.13 33.3]", "DO 18 [AIR KP19]", "DO 19 [STEP DRIVE EN KP20]", "DO 20 [KP21 Y44.1 OPEN]", "DO 21 [ KP22 Y44.1 CLOSE]", "DO 22 [ KP23 Y44.2 OPEN]", "DO 23", "DO 24 [STEP DRIVE 1]", "DO 25 [STEP DRIVE 2]"] ("#DO")
            # "OPEN"
            # "CLOSE"
            # "STOP"
            # "Плавный брос давления в камере\n4.1\tконтроль показаний\n4.2\tконтроль показаний\n5.1\tконтроль показаний\n5.2\tконтроль показаний\n12\t0/1\n18.1\t0/1\n18.2\t0/1\n21\t1\n24\t0/1\n25\t1\n29.1 (33.7)\t0\n29.2 (33.8)\t1\n29.3 (33.9)\t0\n29.4 (33.12)\t0\n29.5 (33.1)\t0\n29.6 (33.2)\t0\n29.7 (33.13)\t0\n29.8 (33.11)\t0\n29.9 (33.10)\t0\n29.10 (33.6)\t0\n29.11 (33.5)\t0\n29.12 (33.4)\t1 -> 0\n29.13 (33.3) \t0\n30\t0\n35.1\t0\n35.2\t0…100%\n36.1\tконтроль показаний\n36.2\tобратная связь\n38.1\tконтроль показаний\n38.2\tконтроль показаний\n38.3\tобратная связь\n41.3\tконтроль показаний\n44.1\t0\n44.2\t0\n46\t0…1,5 В"
            n82 = call "Config Setpoints.vi"("reference in"=w219, "error in (no error)"=w218) -> ("error out"=w217:errorcluster)  [unwired: 13 in]
            n83 = call "DoValve.vi"("reference in"=w246, 5:w222, "error in (no error)"=w217) -> ("reference out"=w250:refnum<class "FPGA API.lvclass">, "error out"=w249:errorcluster)  [unwired: 11 in]
            n84 = call-dynamic "SetHasckelAO.vi"("FPGA API in"=w250, "Haskel in"=0.0, "error in (no error)"=w249) -> ("FPGA API out"=w248:refnum<class "FPGA API.lvclass">, "error out"=w247:errorcluster)  [unwired: 11 in]
            n85 = call-dynamic "SetPropValve.vi"("FPGA API in"=w248, "AO 1"=0.0, "error in (no error)"=w247) -> ("FPGA API out"=w235:refnum<class "FPGA API.lvclass">, "error out"=w234:errorcluster)  [unwired: 11 in]
            n86 = call-dynamic "Enable Close Inlet.vi"("FPGA API in"=w235, "error in (no error)"=w234, "Direction"=Direction."None") -> ("FPGA API out"=w232:refnum<class "FPGA API.lvclass">, "error out"=w231:errorcluster)  [unwired: 11 in]
            n87 = call-dynamic "Enable Close Outlet.vi"("FPGA API in"=w232, "error in (no error)"=w231, "Direction"=Direction."Chamber") -> ("FPGA API out"=w229:refnum<class "FPGA API.lvclass">, "error out"=w228:errorcluster)  [unwired: 11 in]
            n88 = call-dynamic "Enable Stop Step.vi"("FPGA API in"=w229, "error in (no error)"=w228, "Direction"=Direction."Chamber") -> ("error out"=w227:errorcluster)  [unwired: 11 in, 1 out]
            n89 = disable-structure shown="Disabled" {
              disable-tunnel: w238 -> [w254 _]
              disable-tunnel: [w253 _] -> w237
              frame Disabled {
                n90 = call "GetMessageInterface.vi"("Device in"=w254) -> ("MessageInterface"=w252:refnum<class "MessageInterface.lvclass">)  [unwired: 10 in]
                n91 = call-dynamic "SendLocalMsg.vi"("reference in"=w252, "name"="") -> ("error out"=w253:errorcluster)  [unwired: 11 in, 2 out]
              }
              frame Enabled {
              }
            }
            n92 = call "GetMessageInterface.vi"("Device in"=w236) -> ("MessageInterface"=w221:refnum<class "MessageInterface.lvclass">)  [unwired: 10 in]
            n93 = call "Close.vi"("Pump_1AI_1DO_2DI in"=w245) -> ("error out"=w239:errorcluster, "Pump_1AI_1DO_2DI out"=w244:refnum<class "Valve_2DO_2DI.lvclass">)  [unwired: 9 in]
            n94 = call "Close.vi"("Pump_1AI_1DO_2DI in"=w243) -> ("error out"=w240:errorcluster, "Pump_1AI_1DO_2DI out"=w242:refnum<class "Valve_2DO_2DI.lvclass">)  [unwired: 9 in]
            n95 = call-dynamic "SendLocalMsg.vi"("reference in"=w221, "name"="OPEN") -> ("error out"=w225:errorcluster)  [unwired: 11 in, 2 out]
            n96 = Merge Errors(w227, w239, w240, w237, w225) -> (w241:errorcluster)
          }
          frame "Stop Pump" {
            w256 = T7[] [8, 17, 10] items=["DO 0 [KP1] [M12]", "DO 1 [ON KP2] [M21]", "DO 2 [ON KP3] [M24]", "DO 3 [WATER Y18.1 [DO3]]", "DO 4 [WATER Y18.2 [DO4]]", "DO 5 [KP6 Y29.1 33.7]", "DO 6 [KP7 Y29.2 33.8]", "DO 7 [KP8 Y29.3 33.9]", "DO 8 [KP9 Y29.4  33.12]", "DO 9 [KP10 Y29.5 33.1]", "DO 10 [KP11 Y29.6 33.2]", "DO 11 [KP12 Y29.7  33.13]", "DO 12 [KP13 Y29.8  33.11]", "DO 13 [KP14 Y29.9 33.10]", "DO 14 [KP15 Y29.10  33.6]", "DO 15 [KP16 Y29.11  33.5]", "DO 16 [KP17 Y29.12  33.4]", "DO 17 [KP18 Y29.13 33.3]", "DO 18 [AIR KP19]", "DO 19 [STEP DRIVE EN KP20]", "DO 20 [KP21 Y44.1 OPEN]", "DO 21 [ KP22 Y44.1 CLOSE]", "DO 22 [ KP23 Y44.2 OPEN]", "DO 23", "DO 24 [STEP DRIVE 1]", "DO 25 [STEP DRIVE 2]"] ("#DO")
            # "Замер утечек из образца по датчику 41.3\n4.1\tконтроль показаний\n4.2\tконтроль показаний\n5.1\tконтроль показаний\n5.2\tконтроль показаний\n12\t0/1\n18.1\t0/1\n18.2\t0/1\n21\t1\n24\t0/1\n25\t1\n29.1 (33.7)\t0\n29.2 (33.8)\t0\n29.3 (33.9)\t0\n29.4 (33.12)\t1\n29.5 (33.1)\t0\n29.6 (33.2)\t1\n29.7 (33.13)\t0\n29.8 (33.11)\t0\n29.9 (33.10)\t0\n29.10 (33.6)\t0\n29.11 (33.5)\t0\n29.12 (33.4)\t0\n29.13 (33.3) \t1\n30\t0…10 В\n35.1\t60%\n35.2\t0\n36.1\tконтроль показаний\n36.2\tконтроль показаний\n38.1\tконтроль показаний\n38.2\tконтроль показаний\n38.3\tобратная связь\n41.3\tконтроль показаний\n44.1\t0\n44.2\t0\n46\t0…1,5 В"
            # "OPEN"
            # "CLOSE"
            # "STOP"
            n97 = call "Config Setpoints.vi"("reference in"=w259, "error in (no error)"=w258) -> ("error out"=w257:errorcluster)  [unwired: 13 in]
            n98 = call "DoValve.vi"("reference in"=w282, 5:w256, "error in (no error)"=w257) -> ("reference out"=w286:refnum<class "FPGA API.lvclass">, "error out"=w285:errorcluster)  [unwired: 11 in]
            n99 = call-dynamic "SetHasckelAO.vi"("FPGA API in"=w286, "Haskel in"=0.0, "error in (no error)"=w285) -> ("FPGA API out"=w284:refnum<class "FPGA API.lvclass">, "error out"=w283:errorcluster)  [unwired: 11 in]
            n100 = call-dynamic "SetPropValve.vi"("FPGA API in"=w284, "AO 1"=0.0, "error in (no error)"=w283) -> ("FPGA API out"=w271:refnum<class "FPGA API.lvclass">, "error out"=w270:errorcluster)  [unwired: 11 in]
            n101 = call-dynamic "Enable Close Inlet.vi"("FPGA API in"=w271, "error in (no error)"=w270, "Direction"=Direction."None") -> ("FPGA API out"=w268:refnum<class "FPGA API.lvclass">, "error out"=w267:errorcluster)  [unwired: 11 in]
            n102 = call-dynamic "Enable Close Outlet.vi"("FPGA API in"=w268, "error in (no error)"=w267, "Direction"=Direction."None") -> ("FPGA API out"=w265:refnum<class "FPGA API.lvclass">, "error out"=w264:errorcluster)  [unwired: 11 in]
            n103 = call-dynamic "Enable Stop Step.vi"("FPGA API in"=w265, "error in (no error)"=w264, "Direction"=Direction."None") -> ("error out"=w255:errorcluster)  [unwired: 11 in, 1 out]
            n104 = disable-structure shown="Disabled" {
              disable-tunnel: w272 -> [w290 _]
              disable-tunnel: [w289 _] -> w262
              frame Disabled {
                n105 = call "GetMessageInterface.vi"("Device in"=w290) -> ("MessageInterface"=w288:refnum<class "MessageInterface.lvclass">)  [unwired: 10 in]
                n106 = call-dynamic "SendLocalMsg.vi"("reference in"=w288, "name"="OPEN") -> ("error out"=w289:errorcluster)  [unwired: 11 in, 2 out]
              }
              frame Enabled {
              }
            }
            n107 = disable-structure shown="Disabled" {
              disable-tunnel: w274 -> [w294 _]
              disable-tunnel: [w293 _] -> w273
              frame Disabled {
                n108 = call "GetMessageInterface.vi"("Device in"=w294) -> ("MessageInterface"=w292:refnum<class "MessageInterface.lvclass">)  [unwired: 10 in]
                n109 = call-dynamic "SendLocalMsg.vi"("reference in"=w292, "name"="") -> ("error out"=w293:errorcluster)  [unwired: 11 in, 2 out]
              }
              frame Enabled {
              }
            }
            n110 = call "Close.vi"("Pump_1AI_1DO_2DI in"=w281) -> ("error out"=w275:errorcluster, "Pump_1AI_1DO_2DI out"=w280:refnum<class "Valve_2DO_2DI.lvclass">)  [unwired: 9 in]
            n111 = call "Close.vi"("Pump_1AI_1DO_2DI in"=w279) -> ("error out"=w276:errorcluster, "Pump_1AI_1DO_2DI out"=w278:refnum<class "Valve_2DO_2DI.lvclass">)  [unwired: 9 in]
            n112 = Merge Errors(w275, w276, w255, w273, w262) -> (w277:errorcluster)
          }
          frame "IDLE" {
            w299 = T7 1 items=["DO 0 [KP1] [M12]", "DO 1 [ON KP2] [M21]", "DO 2 [ON KP3] [M24]", "DO 3 [WATER Y18.1 [DO3]]", "DO 4 [WATER Y18.2 [DO4]]", "DO 5 [KP6 Y29.1 33.7]", "DO 6 [KP7 Y29.2 33.8]", "DO 7 [KP8 Y29.3 33.9]", "DO 8 [KP9 Y29.4  33.12]", "DO 9 [KP10 Y29.5 33.1]", "DO 10 [KP11 Y29.6 33.2]", "DO 11 [KP12 Y29.7  33.13]", "DO 12 [KP13 Y29.8  33.11]", "DO 13 [KP14 Y29.9 33.10]", "DO 14 [KP15 Y29.10  33.6]", "DO 15 [KP16 Y29.11  33.5]", "DO 16 [KP17 Y29.12  33.4]", "DO 17 [KP18 Y29.13 33.3]", "DO 18 [AIR KP19]", "DO 19 [STEP DRIVE EN KP20]", "DO 20 [KP21 Y44.1 OPEN]", "DO 21 [ KP22 Y44.1 CLOSE]", "DO 22 [ KP23 Y44.2 OPEN]", "DO 23", "DO 24 [STEP DRIVE 1]", "DO 25 [STEP DRIVE 2]"] ("#DO")
            w302 = T7[] [15, 14, 9, 10] items=["DO 0 [KP1] [M12]", "DO 1 [ON KP2] [M21]", "DO 2 [ON KP3] [M24]", "DO 3 [WATER Y18.1 [DO3]]", "DO 4 [WATER Y18.2 [DO4]]", "DO 5 [KP6 Y29.1 33.7]", "DO 6 [KP7 Y29.2 33.8]", "DO 7 [KP8 Y29.3 33.9]", "DO 8 [KP9 Y29.4  33.12]", "DO 9 [KP10 Y29.5 33.1]", "DO 10 [KP11 Y29.6 33.2]", "DO 11 [KP12 Y29.7  33.13]", "DO 12 [KP13 Y29.8  33.11]", "DO 13 [KP14 Y29.9 33.10]", "DO 14 [KP15 Y29.10  33.6]", "DO 15 [KP16 Y29.11  33.5]", "DO 16 [KP17 Y29.12  33.4]", "DO 17 [KP18 Y29.13 33.3]", "DO 18 [AIR KP19]", "DO 19 [STEP DRIVE EN KP20]", "DO 20 [KP21 Y44.1 OPEN]", "DO 21 [ KP22 Y44.1 CLOSE]", "DO 22 [ KP23 Y44.2 OPEN]", "DO 23", "DO 24 [STEP DRIVE 1]", "DO 25 [STEP DRIVE 2]"] ("#DO")
            n113 = call "DoValve.vi"("reference in"=w315, 5:w302, "error in (no error)"=w320) -> ("reference out"=w319:refnum<class "FPGA API.lvclass">, "error out"=w318:errorcluster)  [unwired: 11 in]
            n114 = call-dynamic "SetHasckelAO.vi"("FPGA API in"=w319, "Haskel in"=0.0, "error in (no error)"=w318) -> ("FPGA API out"=w317:refnum<class "FPGA API.lvclass">, "error out"=w316:errorcluster)  [unwired: 11 in]
            n115 = call-dynamic "SetPropValve.vi"("FPGA API in"=w317, "AO 1"=0.0, "error in (no error)"=w316) -> ("FPGA API out"=w312:refnum<class "FPGA API.lvclass">, "error out"=w311:errorcluster)  [unwired: 11 in]
            n116 = call-dynamic "Enable Close Inlet.vi"("FPGA API in"=w312, "error in (no error)"=w311, "Direction"=Direction."None") -> ("FPGA API out"=w309:refnum<class "FPGA API.lvclass">, "error out"=w308:errorcluster)  [unwired: 11 in]
            n117 = call-dynamic "Enable Close Outlet.vi"("FPGA API in"=w309, "error in (no error)"=w308, "Direction"=Direction."None") -> ("FPGA API out"=w306:refnum<class "FPGA API.lvclass">, "error out"=w305:errorcluster)  [unwired: 11 in]
            n118 = call-dynamic "Enable Stop Step.vi"("FPGA API in"=w306, "error in (no error)"=w305, "Direction"=Direction."None") -> ("FPGA API out"=w300:refnum<class "FPGA API.lvclass">, "error out"=w297:errorcluster)  [unwired: 11 in]
            n119 = call-dynamic "Write Do.vi"("FPGA API in"=w300, "#DO"=w299, "value"=FALSE, "Time uSec"=u32 0, "error in (no error)"=w297) -> ("error out"=w296:errorcluster)  [unwired: 9 in, 1 out]
          }
          frame "Filling" {
            w323 = T7[] [10, 5] items=["DO 0 [KP1] [M12]", "DO 1 [ON KP2] [M21]", "DO 2 [ON KP3] [M24]", "DO 3 [WATER Y18.1 [DO3]]", "DO 4 [WATER Y18.2 [DO4]]", "DO 5 [KP6 Y29.1 33.7]", "DO 6 [KP7 Y29.2 33.8]", "DO 7 [KP8 Y29.3 33.9]", "DO 8 [KP9 Y29.4  33.12]", "DO 9 [KP10 Y29.5 33.1]", "DO 10 [KP11 Y29.6 33.2]", "DO 11 [KP12 Y29.7  33.13]", "DO 12 [KP13 Y29.8  33.11]", "DO 13 [KP14 Y29.9 33.10]", "DO 14 [KP15 Y29.10  33.6]", "DO 15 [KP16 Y29.11  33.5]", "DO 16 [KP17 Y29.12  33.4]", "DO 17 [KP18 Y29.13 33.3]", "DO 18 [AIR KP19]", "DO 19 [STEP DRIVE EN KP20]", "DO 20 [KP21 Y44.1 OPEN]", "DO 21 [ KP22 Y44.1 CLOSE]", "DO 22 [ KP23 Y44.2 OPEN]", "DO 23", "DO 24 [STEP DRIVE 1]", "DO 25 [STEP DRIVE 2]"] ("#DO")
            n120 = call "DoValve.vi"("reference in"=w345, 5:w323, "error in (no error)"=w350) -> ("reference out"=w349:refnum<class "FPGA API.lvclass">, "error out"=w348:errorcluster)  [unwired: 11 in]
            n121 = call-dynamic "SetHasckelAO.vi"("FPGA API in"=w349, "Haskel in"=0.0, "error in (no error)"=w348) -> ("FPGA API out"=w347:refnum<class "FPGA API.lvclass">, "error out"=w346:errorcluster)  [unwired: 11 in]
            n122 = call-dynamic "SetPropValve.vi"("FPGA API in"=w347, "AO 1"=0.0, "error in (no error)"=w346) -> ("FPGA API out"=w334:refnum<class "FPGA API.lvclass">, "error out"=w333:errorcluster)  [unwired: 11 in]
            n123 = call-dynamic "Enable Close Inlet.vi"("FPGA API in"=w334, "error in (no error)"=w333, "Direction"=Direction."None") -> ("FPGA API out"=w331:refnum<class "FPGA API.lvclass">, "error out"=w330:errorcluster)  [unwired: 11 in]
            n124 = call-dynamic "Enable Close Outlet.vi"("FPGA API in"=w331, "error in (no error)"=w330, "Direction"=Direction."None") -> ("FPGA API out"=w328:refnum<class "FPGA API.lvclass">, "error out"=w327:errorcluster)  [unwired: 11 in]
            n125 = call-dynamic "Enable Stop Step.vi"("FPGA API in"=w328, "error in (no error)"=w327, "Direction"=Direction."None") -> ("error out"=w326:errorcluster)  [unwired: 11 in, 1 out]
            n126 = disable-structure shown="Disabled" {
              disable-tunnel: w337 -> [w358 _]
              disable-tunnel: [w356 _] -> w336
              disable-tunnel: w335 -> [w354 _]
              disable-tunnel: [w351 _] -> w324
              frame Disabled {
                # "OPEN"
                # "CLOSE"
                # "STOP"
                n127 = call "GetMessageInterface.vi"("Device in"=w354) -> ("MessageInterface"=w355:refnum<class "MessageInterface.lvclass">)  [unwired: 10 in]
                n128 = call "GetMessageInterface.vi"("Device in"=w358) -> ("MessageInterface"=w357:refnum<class "MessageInterface.lvclass">)  [unwired: 10 in]
                n129 = call-dynamic "SendLocalMsg.vi"("reference in"=w355, "name"="") -> ("error out"=w351:errorcluster)  [unwired: 11 in, 2 out]
                n130 = call-dynamic "SendLocalMsg.vi"("reference in"=w357, "name"="") -> ("error out"=w356:errorcluster)  [unwired: 11 in, 2 out]
              }
              frame Enabled {
              }
            }
            n131 = call "Close.vi"("Pump_1AI_1DO_2DI in"=w344) -> ("error out"=w338:errorcluster, "Pump_1AI_1DO_2DI out"=w343:refnum<class "Valve_2DO_2DI.lvclass">)  [unwired: 9 in]
            n132 = call "Close.vi"("Pump_1AI_1DO_2DI in"=w342) -> ("error out"=w339:errorcluster, "Pump_1AI_1DO_2DI out"=w341:refnum<class "Valve_2DO_2DI.lvclass">)  [unwired: 9 in]
            n133 = Merge Errors(w326, w338, w339, w336, w324) -> (w340:errorcluster)
          }
          frame "Low Pressure" {
            w361 = T7[] [9, 5] items=["DO 0 [KP1] [M12]", "DO 1 [ON KP2] [M21]", "DO 2 [ON KP3] [M24]", "DO 3 [WATER Y18.1 [DO3]]", "DO 4 [WATER Y18.2 [DO4]]", "DO 5 [KP6 Y29.1 33.7]", "DO 6 [KP7 Y29.2 33.8]", "DO 7 [KP8 Y29.3 33.9]", "DO 8 [KP9 Y29.4  33.12]", "DO 9 [KP10 Y29.5 33.1]", "DO 10 [KP11 Y29.6 33.2]", "DO 11 [KP12 Y29.7  33.13]", "DO 12 [KP13 Y29.8  33.11]", "DO 13 [KP14 Y29.9 33.10]", "DO 14 [KP15 Y29.10  33.6]", "DO 15 [KP16 Y29.11  33.5]", "DO 16 [KP17 Y29.12  33.4]", "DO 17 [KP18 Y29.13 33.3]", "DO 18 [AIR KP19]", "DO 19 [STEP DRIVE EN KP20]", "DO 20 [KP21 Y44.1 OPEN]", "DO 21 [ KP22 Y44.1 CLOSE]", "DO 22 [ KP23 Y44.2 OPEN]", "DO 23", "DO 24 [STEP DRIVE 1]", "DO 25 [STEP DRIVE 2]"] ("#DO")
            n134 = call "DoValve.vi"("reference in"=w383, 5:w361, "error in (no error)"=w388) -> ("reference out"=w387:refnum<class "FPGA API.lvclass">, "error out"=w386:errorcluster)  [unwired: 11 in]
            n135 = call-dynamic "SetHasckelAO.vi"("FPGA API in"=w387, "Haskel in"=0.0, "error in (no error)"=w386) -> ("FPGA API out"=w385:refnum<class "FPGA API.lvclass">, "error out"=w384:errorcluster)  [unwired: 11 in]
            n136 = call-dynamic "SetPropValve.vi"("FPGA API in"=w385, "AO 1"=0.0, "error in (no error)"=w384) -> ("FPGA API out"=w372:refnum<class "FPGA API.lvclass">, "error out"=w371:errorcluster)  [unwired: 11 in]
            n137 = call-dynamic "Enable Close Inlet.vi"("FPGA API in"=w372, "error in (no error)"=w371, "Direction"=Direction."None") -> ("FPGA API out"=w369:refnum<class "FPGA API.lvclass">, "error out"=w368:errorcluster)  [unwired: 11 in]
            n138 = call-dynamic "Enable Close Outlet.vi"("FPGA API in"=w369, "error in (no error)"=w368, "Direction"=Direction."None") -> ("FPGA API out"=w366:refnum<class "FPGA API.lvclass">, "error out"=w365:errorcluster)  [unwired: 11 in]
            n139 = call-dynamic "Enable Stop Step.vi"("FPGA API in"=w366, "error in (no error)"=w365, "Direction"=Direction."None") -> ("error out"=w364:errorcluster)  [unwired: 11 in, 1 out]
            n140 = disable-structure shown="Disabled" {
              disable-tunnel: w375 -> [w396 _]
              disable-tunnel: [w394 _] -> w374
              disable-tunnel: w373 -> [w392 _]
              disable-tunnel: [w389 _] -> w362
              frame Disabled {
                # "OPEN"
                # "CLOSE"
                # "STOP"
                n141 = call "GetMessageInterface.vi"("Device in"=w392) -> ("MessageInterface"=w393:refnum<class "MessageInterface.lvclass">)  [unwired: 10 in]
                n142 = call "GetMessageInterface.vi"("Device in"=w396) -> ("MessageInterface"=w395:refnum<class "MessageInterface.lvclass">)  [unwired: 10 in]
                n143 = call-dynamic "SendLocalMsg.vi"("reference in"=w393, "name"="") -> ("error out"=w389:errorcluster)  [unwired: 11 in, 2 out]
                n144 = call-dynamic "SendLocalMsg.vi"("reference in"=w395, "name"="") -> ("error out"=w394:errorcluster)  [unwired: 11 in, 2 out]
              }
              frame Enabled {
              }
            }
            n145 = call "Close.vi"("Pump_1AI_1DO_2DI in"=w382) -> ("error out"=w376:errorcluster, "Pump_1AI_1DO_2DI out"=w381:refnum<class "Valve_2DO_2DI.lvclass">)  [unwired: 9 in]
            n146 = call "Close.vi"("Pump_1AI_1DO_2DI in"=w380) -> ("error out"=w377:errorcluster, "Pump_1AI_1DO_2DI out"=w379:refnum<class "Valve_2DO_2DI.lvclass">)  [unwired: 9 in]
            n147 = Merge Errors(w364, w376, w377, w374, w362) -> (w378:errorcluster)
          }
          frame "Hi Pressure" {
            w399 = T7[] [5] items=["DO 0 [KP1] [M12]", "DO 1 [ON KP2] [M21]", "DO 2 [ON KP3] [M24]", "DO 3 [WATER Y18.1 [DO3]]", "DO 4 [WATER Y18.2 [DO4]]", "DO 5 [KP6 Y29.1 33.7]", "DO 6 [KP7 Y29.2 33.8]", "DO 7 [KP8 Y29.3 33.9]", "DO 8 [KP9 Y29.4  33.12]", "DO 9 [KP10 Y29.5 33.1]", "DO 10 [KP11 Y29.6 33.2]", "DO 11 [KP12 Y29.7  33.13]", "DO 12 [KP13 Y29.8  33.11]", "DO 13 [KP14 Y29.9 33.10]", "DO 14 [KP15 Y29.10  33.6]", "DO 15 [KP16 Y29.11  33.5]", "DO 16 [KP17 Y29.12  33.4]", "DO 17 [KP18 Y29.13 33.3]", "DO 18 [AIR KP19]", "DO 19 [STEP DRIVE EN KP20]", "DO 20 [KP21 Y44.1 OPEN]", "DO 21 [ KP22 Y44.1 CLOSE]", "DO 22 [ KP23 Y44.2 OPEN]", "DO 23", "DO 24 [STEP DRIVE 1]", "DO 25 [STEP DRIVE 2]"] ("#DO")
            n148 = call "DoValve.vi"("reference in"=w421, 5:w399, "error in (no error)"=w426) -> ("reference out"=w425:refnum<class "FPGA API.lvclass">, "error out"=w424:errorcluster)  [unwired: 11 in]
            n149 = call-dynamic "SetHasckelAO.vi"("FPGA API in"=w425, "Haskel in"=0.0, "error in (no error)"=w424) -> ("FPGA API out"=w423:refnum<class "FPGA API.lvclass">, "error out"=w422:errorcluster)  [unwired: 11 in]
            n150 = call-dynamic "SetPropValve.vi"("FPGA API in"=w423, "AO 1"=0.0, "error in (no error)"=w422) -> ("FPGA API out"=w410:refnum<class "FPGA API.lvclass">, "error out"=w409:errorcluster)  [unwired: 11 in]
            n151 = call-dynamic "Enable Close Inlet.vi"("FPGA API in"=w410, "error in (no error)"=w409, "Direction"=Direction."None") -> ("FPGA API out"=w407:refnum<class "FPGA API.lvclass">, "error out"=w406:errorcluster)  [unwired: 11 in]
            n152 = call-dynamic "Enable Close Outlet.vi"("FPGA API in"=w407, "error in (no error)"=w406, "Direction"=Direction."None") -> ("FPGA API out"=w404:refnum<class "FPGA API.lvclass">, "error out"=w403:errorcluster)  [unwired: 11 in]
            n153 = call-dynamic "Enable Stop Step.vi"("FPGA API in"=w404, "error in (no error)"=w403, "Direction"=Direction."None") -> ("error out"=w402:errorcluster)  [unwired: 11 in, 1 out]
            n154 = disable-structure shown="Disabled" {
              disable-tunnel: w413 -> [w434 _]
              disable-tunnel: [w432 _] -> w412
              disable-tunnel: w411 -> [w430 _]
              disable-tunnel: [w427 _] -> w400
              frame Disabled {
                # "OPEN"
                # "CLOSE"
                # "STOP"
                n155 = call "GetMessageInterface.vi"("Device in"=w430) -> ("MessageInterface"=w431:refnum<class "MessageInterface.lvclass">)  [unwired: 10 in]
                n156 = call "GetMessageInterface.vi"("Device in"=w434) -> ("MessageInterface"=w433:refnum<class "MessageInterface.lvclass">)  [unwired: 10 in]
                n157 = call-dynamic "SendLocalMsg.vi"("reference in"=w431, "name"="") -> ("error out"=w427:errorcluster)  [unwired: 11 in, 2 out]
                n158 = call-dynamic "SendLocalMsg.vi"("reference in"=w433, "name"="") -> ("error out"=w432:errorcluster)  [unwired: 11 in, 2 out]
              }
              frame Enabled {
              }
            }
            n159 = call "Close.vi"("Pump_1AI_1DO_2DI in"=w420) -> ("error out"=w414:errorcluster, "Pump_1AI_1DO_2DI out"=w419:refnum<class "Valve_2DO_2DI.lvclass">)  [unwired: 9 in]
            n160 = call "Close.vi"("Pump_1AI_1DO_2DI in"=w418) -> ("error out"=w415:errorcluster, "Pump_1AI_1DO_2DI out"=w417:refnum<class "Valve_2DO_2DI.lvclass">)  [unwired: 9 in]
            n161 = Merge Errors(w402, w414, w415, w412, w400) -> (w416:errorcluster)
          }
          frame "Abrupt Pressure Release" {
            w435 = T7[] [8, 17, 10] items=["DO 0 [KP1] [M12]", "DO 1 [ON KP2] [M21]", "DO 2 [ON KP3] [M24]", "DO 3 [WATER Y18.1 [DO3]]", "DO 4 [WATER Y18.2 [DO4]]", "DO 5 [KP6 Y29.1 33.7]", "DO 6 [KP7 Y29.2 33.8]", "DO 7 [KP8 Y29.3 33.9]", "DO 8 [KP9 Y29.4  33.12]", "DO 9 [KP10 Y29.5 33.1]", "DO 10 [KP11 Y29.6 33.2]", "DO 11 [KP12 Y29.7  33.13]", "DO 12 [KP13 Y29.8  33.11]", "DO 13 [KP14 Y29.9 33.10]", "DO 14 [KP15 Y29.10  33.6]", "DO 15 [KP16 Y29.11  33.5]", "DO 16 [KP17 Y29.12  33.4]", "DO 17 [KP18 Y29.13 33.3]", "DO 18 [AIR KP19]", "DO 19 [STEP DRIVE EN KP20]", "DO 20 [KP21 Y44.1 OPEN]", "DO 21 [ KP22 Y44.1 CLOSE]", "DO 22 [ KP23 Y44.2 OPEN]", "DO 23", "DO 24 [STEP DRIVE 1]", "DO 25 [STEP DRIVE 2]"] ("#DO")
            # "Замер утечек из образца по датчику 41.3\n4.1\tконтроль показаний\n4.2\tконтроль показаний\n5.1\tконтроль показаний\n5.2\tконтроль показаний\n12\t0/1\n18.1\t0/1\n18.2\t0/1\n21\t1\n24\t0/1\n25\t1\n29.1 (33.7)\t0\n29.2 (33.8)\t0\n29.3 (33.9)\t0\n29.4 (33.12)\t1\n29.5 (33.1)\t0\n29.6 (33.2)\t1\n29.7 (33.13)\t0\n29.8 (33.11)\t0\n29.9 (33.10)\t0\n29.10 (33.6)\t0\n29.11 (33.5)\t0\n29.12 (33.4)\t0\n29.13 (33.3) \t1\n30\t0…10 В\n35.1\t60%\n35.2\t0\n36.1\tконтроль показаний\n36.2\tконтроль показаний\n38.1\tконтроль показаний\n38.2\tконтроль показаний\n38.3\tобратная связь\n41.3\tконтроль показаний\n44.1\t0\n44.2\t0\n46\t0…1,5 В"
            # "OPEN"
            # "CLOSE"
            # "STOP"
            n162 = Unbundle By Name(w462) -> ("Pressure SP"=w440:dbl)
            n163 = call "Config Setpoints.vi"("reference in"=w438, "error in (no error)"=w437) -> ("error out"=w436:errorcluster)  [unwired: 13 in]
            n164 = call "Pressure to voltage.vi"("Pressure SP"=w440) -> ()  [unwired: 14 in, 1 out]
            n165 = call "DoValve.vi"("reference in"=w464, 5:w435, "error in (no error)"=w436) -> ("reference out"=w468:refnum<class "FPGA API.lvclass">, "error out"=w467:errorcluster)  [unwired: 11 in]
            n166 = call-dynamic "SetHasckelAO.vi"("FPGA API in"=w468, "Haskel in"=0.0, "error in (no error)"=w467) -> ("FPGA API out"=w466:refnum<class "FPGA API.lvclass">, "error out"=w465:errorcluster)  [unwired: 11 in]
            n167 = call-dynamic "SetPropValve.vi"("FPGA API in"=w466, "AO 1"=0.0, "error in (no error)"=w465) -> ("FPGA API out"=w452:refnum<class "FPGA API.lvclass">, "error out"=w451:errorcluster)  [unwired: 11 in]
            n168 = call-dynamic "Enable Close Inlet.vi"("FPGA API in"=w452, "error in (no error)"=w451, "Direction"=Direction."None") -> ("FPGA API out"=w449:refnum<class "FPGA API.lvclass">, "error out"=w448:errorcluster)  [unwired: 11 in]
            n169 = call-dynamic "Enable Close Outlet.vi"("FPGA API in"=w449, "error in (no error)"=w448, "Direction"=Direction."None") -> ("FPGA API out"=w446:refnum<class "FPGA API.lvclass">, "error out"=w445:errorcluster)  [unwired: 11 in]
            n170 = call-dynamic "Enable Stop Step.vi"("FPGA API in"=w446, "error in (no error)"=w445, "Direction"=Direction."None") -> ("error out"=w444:errorcluster)  [unwired: 11 in, 1 out]
            n171 = disable-structure shown="Disabled" {
              disable-tunnel: w455 -> [w476 _]
              disable-tunnel: [w475 _] -> w454
              frame Disabled {
                n172 = call "GetMessageInterface.vi"("Device in"=w476) -> ("MessageInterface"=w474:refnum<class "MessageInterface.lvclass">)  [unwired: 10 in]
                n173 = call-dynamic "SendLocalMsg.vi"("reference in"=w474, "name"="") -> ("error out"=w475:errorcluster)  [unwired: 11 in, 2 out]
              }
              frame Enabled {
              }
            }
            n174 = disable-structure shown="Disabled" {
              disable-tunnel: w453 -> [w472 _]
              disable-tunnel: [w471 _] -> w442
              frame Disabled {
                n175 = call "GetMessageInterface.vi"("Device in"=w472) -> ("MessageInterface"=w470:refnum<class "MessageInterface.lvclass">)  [unwired: 10 in]
                n176 = call-dynamic "SendLocalMsg.vi"("reference in"=w470, "name"="OPEN") -> ("error out"=w471:errorcluster)  [unwired: 11 in, 2 out]
              }
              frame Enabled {
              }
            }
            n177 = call "Close.vi"("Pump_1AI_1DO_2DI in"=w463) -> ("error out"=w456:errorcluster, "Pump_1AI_1DO_2DI out"=w461:refnum<class "Valve_2DO_2DI.lvclass">)  [unwired: 9 in]
            n178 = call "Close.vi"("Pump_1AI_1DO_2DI in"=w460) -> ("error out"=w457:errorcluster, "Pump_1AI_1DO_2DI out"=w459:refnum<class "Valve_2DO_2DI.lvclass">)  [unwired: 9 in]
            n179 = Merge Errors(w444, w456, w457, w454, w442) -> (w458:errorcluster)
          }
          frame "Smooth Pressure Release" {
            w484 = T8 7 items=["AI 0 Cooling Station Level", "AI 1 Cooling Station Temp", "AI 2 Oil Supply Level", "AI 3 Oil Supply Temp", "AI 4 ", "AI 5 Pressure Haskel", "AI 6 Pressure DUT", "AI 7 Pressure Chamber", "AI 8 Pressure Air inlet", "AI 9 Pressure Air outlet", "AI 10 Pressure Messure Line"] ("AI index")
            w492 = T7[] [16, 7] items=["DO 0 [KP1] [M12]", "DO 1 [ON KP2] [M21]", "DO 2 [ON KP3] [M24]", "DO 3 [WATER Y18.1 [DO3]]", "DO 4 [WATER Y18.2 [DO4]]", "DO 5 [KP6 Y29.1 33.7]", "DO 6 [KP7 Y29.2 33.8]", "DO 7 [KP8 Y29.3 33.9]", "DO 8 [KP9 Y29.4  33.12]", "DO 9 [KP10 Y29.5 33.1]", "DO 10 [KP11 Y29.6 33.2]", "DO 11 [KP12 Y29.7  33.13]", "DO 12 [KP13 Y29.8  33.11]", "DO 13 [KP14 Y29.9 33.10]", "DO 14 [KP15 Y29.10  33.6]", "DO 15 [KP16 Y29.11  33.5]", "DO 16 [KP17 Y29.12  33.4]", "DO 17 [KP18 Y29.13 33.3]", "DO 18 [AIR KP19]", "DO 19 [STEP DRIVE EN KP20]", "DO 20 [KP21 Y44.1 OPEN]", "DO 21 [ KP22 Y44.1 CLOSE]", "DO 22 [ KP23 Y44.2 OPEN]", "DO 23", "DO 24 [STEP DRIVE 1]", "DO 25 [STEP DRIVE 2]"] ("#DO")
            n180 = Unbundle By Name(w482) -> ("AIs"=w483:refnum<class "AI.lvclass">[])
            n181 = Unbundle By Name(w482) -> ("ExpFitter_DUT"=w487:refnum<class "ExpFitter.lvclass">, "Pressure SP"=w481:dbl)
            n182 = call "Config Setpoints.vi"("reference in"=w490, "error in (no error)"=w489) -> ("error out"=w488:errorcluster)  [unwired: 13 in]
            n183 = Index Array(array=w483, index=w484) -> (element=w485:refnum<class "AI.lvclass">)
            n184 = call "Get_Values.vi"("reference in"=w485) -> ("Data"=w486:T9)  [unwired: 14 in]
            n185 = Unbundle By Name(w486) -> ("Stat Data.scl mean 1Hz"=w480:dbl)
            n186 = call "Calc Time.vi"("SP"=w481, "PV"=w480, "ExpFitter in"=w487) -> ("dT"=w479:dbl)  [unwired: 6 in, 2 out]
            n187 = Multiply(x=w479, y=1000000.0) -> (x*y=w477:dbl)
            n188 = call "DoValve.vi"("reference in"=w506, 5:w492, 7:w477, "error in (no error)"=w488) -> ("reference out"=w510:refnum<class "FPGA API.lvclass">, "error out"=w509:errorcluster)  [unwired: 10 in]
            n189 = call-dynamic "SetHasckelAO.vi"("FPGA API in"=w510, "Haskel in"=0.0, "error in (no error)"=w509) -> ("FPGA API out"=w508:refnum<class "FPGA API.lvclass">, "error out"=w507:errorcluster)  [unwired: 11 in]
            n190 = call-dynamic "SetPropValve.vi"("FPGA API in"=w508, "AO 1"=0.0, "error in (no error)"=w507) -> ("FPGA API out"=w503:refnum<class "FPGA API.lvclass">, "error out"=w502:errorcluster)  [unwired: 11 in]
            n191 = call-dynamic "Enable Close Inlet.vi"("FPGA API in"=w503, "error in (no error)"=w502, "Direction"=Direction."None") -> ("FPGA API out"=w500:refnum<class "FPGA API.lvclass">, "error out"=w499:errorcluster)  [unwired: 11 in]
            n192 = call-dynamic "Enable Close Outlet.vi"("FPGA API in"=w500, "error in (no error)"=w499, "Direction"=Direction."None") -> ("FPGA API out"=w497:refnum<class "FPGA API.lvclass">, "error out"=w496:errorcluster)  [unwired: 11 in]
            n193 = call-dynamic "Enable Stop Step.vi"("FPGA API in"=w497, "error in (no error)"=w496, "Direction"=Direction."None") -> ("error out"=w495:errorcluster)  [unwired: 11 in, 1 out]
          }
          frame "Measuring Leakage Sensor 41.3" {
            w518 = T8 6 items=["AI 0 Cooling Station Level", "AI 1 Cooling Station Temp", "AI 2 Oil Supply Level", "AI 3 Oil Supply Temp", "AI 4 ", "AI 5 Pressure Haskel", "AI 6 Pressure DUT", "AI 7 Pressure Chamber", "AI 8 Pressure Air inlet", "AI 9 Pressure Air outlet", "AI 10 Pressure Messure Line"] ("AI index")
            w526 = T7[] [17, 6] items=["DO 0 [KP1] [M12]", "DO 1 [ON KP2] [M21]", "DO 2 [ON KP3] [M24]", "DO 3 [WATER Y18.1 [DO3]]", "DO 4 [WATER Y18.2 [DO4]]", "DO 5 [KP6 Y29.1 33.7]", "DO 6 [KP7 Y29.2 33.8]", "DO 7 [KP8 Y29.3 33.9]", "DO 8 [KP9 Y29.4  33.12]", "DO 9 [KP10 Y29.5 33.1]", "DO 10 [KP11 Y29.6 33.2]", "DO 11 [KP12 Y29.7  33.13]", "DO 12 [KP13 Y29.8  33.11]", "DO 13 [KP14 Y29.9 33.10]", "DO 14 [KP15 Y29.10  33.6]", "DO 15 [KP16 Y29.11  33.5]", "DO 16 [KP17 Y29.12  33.4]", "DO 17 [KP18 Y29.13 33.3]", "DO 18 [AIR KP19]", "DO 19 [STEP DRIVE EN KP20]", "DO 20 [KP21 Y44.1 OPEN]", "DO 21 [ KP22 Y44.1 CLOSE]", "DO 22 [ KP23 Y44.2 OPEN]", "DO 23", "DO 24 [STEP DRIVE 1]", "DO 25 [STEP DRIVE 2]"] ("#DO")
            n194 = Unbundle By Name(w516) -> ("AIs"=w517:refnum<class "AI.lvclass">[])
            n195 = Unbundle By Name(w516) -> ("ExpFitter_DUT"=w521:refnum<class "ExpFitter.lvclass">, "Pressure SP"=w515:dbl)
            n196 = call "Config Setpoints.vi"("reference in"=w524, "error in (no error)"=w523) -> ("error out"=w522:errorcluster)  [unwired: 13 in]
            n197 = Index Array(array=w517, index=w518) -> (element=w519:refnum<class "AI.lvclass">)
            n198 = call "Get_Values.vi"("reference in"=w519) -> ("Data"=w520:T9)  [unwired: 14 in]
            n199 = Unbundle By Name(w520) -> ("Stat Data.scl mean 1Hz"=w514:dbl)
            n200 = call "Calc Time.vi"("SP"=w515, "PV"=w514, "ExpFitter in"=w521) -> ("dT"=w513:dbl)  [unwired: 6 in, 2 out]
            n201 = Multiply(x=w513, y=1000000.0) -> (x*y=w511:dbl)
            n202 = call "DoValve.vi"("reference in"=w540, 5:w526, 7:w511, "error in (no error)"=w522) -> ("reference out"=w544:refnum<class "FPGA API.lvclass">, "error out"=w543:errorcluster)  [unwired: 10 in]
            n203 = call-dynamic "SetHasckelAO.vi"("FPGA API in"=w544, "Haskel in"=0.0, "error in (no error)"=w543) -> ("FPGA API out"=w542:refnum<class "FPGA API.lvclass">, "error out"=w541:errorcluster)  [unwired: 11 in]
            n204 = call-dynamic "SetPropValve.vi"("FPGA API in"=w542, "AO 1"=0.0, "error in (no error)"=w541) -> ("FPGA API out"=w537:refnum<class "FPGA API.lvclass">, "error out"=w536:errorcluster)  [unwired: 11 in]
            n205 = call-dynamic "Enable Close Inlet.vi"("FPGA API in"=w537, "error in (no error)"=w536, "Direction"=Direction."None") -> ("FPGA API out"=w534:refnum<class "FPGA API.lvclass">, "error out"=w533:errorcluster)  [unwired: 11 in]
            n206 = call-dynamic "Enable Close Outlet.vi"("FPGA API in"=w534, "error in (no error)"=w533, "Direction"=Direction."None") -> ("FPGA API out"=w531:refnum<class "FPGA API.lvclass">, "error out"=w530:errorcluster)  [unwired: 11 in]
            n207 = call-dynamic "Enable Stop Step.vi"("FPGA API in"=w531, "error in (no error)"=w530, "Direction"=Direction."None") -> ("error out"=w529:errorcluster)  [unwired: 11 in, 1 out]
          }
          frame "Measuring Leakage Burette 42" {
            w546 = T7 18 items=["DO 0 [KP1] [M12]", "DO 1 [ON KP2] [M21]", "DO 2 [ON KP3] [M24]", "DO 3 [WATER Y18.1 [DO3]]", "DO 4 [WATER Y18.2 [DO4]]", "DO 5 [KP6 Y29.1 33.7]", "DO 6 [KP7 Y29.2 33.8]", "DO 7 [KP8 Y29.3 33.9]", "DO 8 [KP9 Y29.4  33.12]", "DO 9 [KP10 Y29.5 33.1]", "DO 10 [KP11 Y29.6 33.2]", "DO 11 [KP12 Y29.7  33.13]", "DO 12 [KP13 Y29.8  33.11]", "DO 13 [KP14 Y29.9 33.10]", "DO 14 [KP15 Y29.10  33.6]", "DO 15 [KP16 Y29.11  33.5]", "DO 16 [KP17 Y29.12  33.4]", "DO 17 [KP18 Y29.13 33.3]", "DO 18 [AIR KP19]", "DO 19 [STEP DRIVE EN KP20]", "DO 20 [KP21 Y44.1 OPEN]", "DO 21 [ KP22 Y44.1 CLOSE]", "DO 22 [ KP23 Y44.2 OPEN]", "DO 23", "DO 24 [STEP DRIVE 1]", "DO 25 [STEP DRIVE 2]"] ("DO index")
            n208 = call-dynamic "Write Do.vi"("FPGA API in"=w550, "#DO"=w546, "value"=TRUE, "Time uSec"=u32 0, "error in (no error)"=w549) -> ("FPGA API out"=w547:refnum<class "FPGA API.lvclass">, "error out"=w548:errorcluster)  [unwired: 9 in]
            n209 = call-dynamic "SetHasckelAO.vi"("FPGA API in"=w547, "Haskel in"=0.0, "error in (no error)"=w548) -> ("FPGA API out"=w572:refnum<class "FPGA API.lvclass">, "error out"=w571:errorcluster)  [unwired: 11 in]
            n210 = call-dynamic "SetPropValve.vi"("FPGA API in"=w572, "AO 1"=0.0, "error in (no error)"=w571) -> ("FPGA API out"=w564:refnum<class "FPGA API.lvclass">, "error out"=w563:errorcluster)  [unwired: 11 in]
            n211 = call-dynamic "Enable Close Inlet.vi"("FPGA API in"=w564, "error in (no error)"=w563, "Direction"=Direction."None") -> ("FPGA API out"=w561:refnum<class "FPGA API.lvclass">, "error out"=w560:errorcluster)  [unwired: 11 in]
            n212 = call-dynamic "Enable Close Outlet.vi"("FPGA API in"=w561, "error in (no error)"=w560, "Direction"=Direction."None") -> ("FPGA API out"=w558:refnum<class "FPGA API.lvclass">, "error out"=w557:errorcluster)  [unwired: 11 in]
            n213 = call-dynamic "Enable Stop Step.vi"("FPGA API in"=w558, "error in (no error)"=w557, "Direction"=Direction."None") -> ("error out"=w545:errorcluster)  [unwired: 11 in, 1 out]
            n214 = disable-structure shown="Disabled" {
              disable-tunnel: w567 -> [w580 _]
              disable-tunnel: [w578 _] -> w566
              disable-tunnel: w565 -> [w576 _]
              disable-tunnel: [w573 _] -> w555
              frame Disabled {
                # "OPEN"
                # "CLOSE"
                # "STOP"
                n215 = call "GetMessageInterface.vi"("Device in"=w576) -> ("MessageInterface"=w577:refnum<class "MessageInterface.lvclass">)  [unwired: 10 in]
                n216 = call "GetMessageInterface.vi"("Device in"=w580) -> ("MessageInterface"=w579:refnum<class "MessageInterface.lvclass">)  [unwired: 10 in]
                n217 = call-dynamic "SendLocalMsg.vi"("reference in"=w577, "name"="") -> ("error out"=w573:errorcluster)  [unwired: 11 in, 2 out]
                n218 = call-dynamic "SendLocalMsg.vi"("reference in"=w579, "name"="") -> ("error out"=w578:errorcluster)  [unwired: 11 in, 2 out]
              }
              frame Enabled {
              }
            }
            n219 = Merge Errors(w545, w566, w555) -> (w568:errorcluster)
          }
        }
        n220 = in-place-cluster #1("VLV 44.1"=w20, "VLV 44.2"=w19) -> (w12:refnum<class "Stand.lvclass">)
      }
    }
    frame False {
      n221 = in-place {
        in-place-border: [w598] -> w581
        in-place-border: w584 -> [w597]
        in-place-border: w583 -> [w587]
        n222 = in-place-cluster #2(w583) -> ("MODE"=w585:T1, "PM"=w595:refnum<class "PM_Group.lvclass">, "VLV 44.1"=w594:refnum<class "Valve_2DO_2DI.lvclass">, "VLV 44.2"=w593:refnum<class "Valve_2DO_2DI.lvclass">)
        n223 = Unbundle By Name(w587) -> ("NV_DUT"=w589:refnum<class "NeedleValve.lvclass">, "NV_Chamber"=w588:refnum<class "NeedleValve.lvclass">)
        n224 = call "GetFPGA.vi"("Device in"=w587) -> ("FPGA API.lvclass"=w596:refnum<class "FPGA API.lvclass">)  [unwired: 10 in]
        n225 = case shown="\"Low Pressure DUT\"" w585 {
          selector: w585 -> [w599 w610 w642 w675 _ _ _ _ _ _ w731 w825 w852 _ w878 w893 w898 w940 w948 w956]
          tunnel: w597 -> [w603 w606 w638 w678 w692 w697 w702 w706 w720 w725 w732 w814 w855 w869 w881 w894 w901 w943 w951 w959]
          tunnel: [w603 w605 w637 w669 w692 w697 w702 w704 w720 w725 w729 w815 w846 w869 w871 w894 w924 w944 w952 w960] -> w598
          tunnel: w594 -> [w601 w623 w655 w682 w691 w696 w701 w710 w719 w724 w736 w829 w859 w868 w885 w896 w930 w947 w955 w963]
          tunnel: w593 -> [w600 w622 w654 w680 w689 w694 w699 w709 w717 w722 w734 w827 w857 w866 w883 w895 w926 w945 w953 w961]
          tunnel: w596 -> [_ _ _ w679 _ _ _ _ _ _ w733 w816 w856 _ w882 _ w931 _ _ _]
          tunnel: w595 -> [w602 w608 w640 w681 w690 w695 w700 w707 w718 w723 w735 w828 w858 w867 w884 w897 w929 w946 w954 w962]
          tunnel: [w602 w607 w639 w681 w690 w695 w700 w705 w718 w723 w735 w828 w858 w867 w884 w897 w929 w946 w954 w962] -> w592
          tunnel: w587 -> [_ w616 w648 w671 _ _ _ _ _ _ w728 w822 _ _ w873 _ w928 _ _ _]
          tunnel: [w601 w623 w655 w682 w691 w696 w701 w710 w719 w724 w736 w829 w859 w868 w885 w896 w927 w947 w955 w963] -> w591
          tunnel: [w600 w622 w654 w680 w689 w694 w699 w709 w717 w722 w734 w827 w857 w866 w883 w895 w925 w945 w953 w961] -> w590
          tunnel: w589 -> [_ _ _ _ _ _ _ _ _ _ w727 _ _ _ _ _ w921 _ _ _]
          tunnel: w588 -> [_ _ _ _ _ _ _ _ _ _ _ _ _ _ _ _ w919 _ _ _]
          tunnel: w587 -> [_ w617 w649 _ _ _ _ _ _ _ w726 w826 _ _ _ _ w902 w941 w949 w957]
          tunnel: [w599 w609 w641 w672 Step_Name."IDLE" ("stepName") Step_Name."IDLE" ("stepName") Step_Name."IDLE" ("stepName") Step_Name."NONE" ("STEP") Step_Name."IDLE" ("stepName") Step_Name."IDLE" ("stepName") w730 w825 w848 Step_Name."IDLE" ("stepName") w874 w893 w898 w940 w948 w956] -> w586
          frame "IDLE" {
          }
          frame "Filling" {
            w619 = T8 0 items=["AI 0 Cooling Station Level", "AI 1 Cooling Station Temp", "AI 2 Oil Supply Level", "AI 3 Oil Supply Temp", "AI 4 ", "AI 5 Pressure Haskel", "AI 6 Pressure DUT", "AI 7 Pressure Chamber", "AI 8 Pressure Air inlet", "AI 9 Pressure Air outlet", "AI 10 Pressure Messure Line"] ("AI index")
            n226 = Unbundle By Name(w616) -> ("Filling Delta Level [%]"=w615:dbl, "BeginFilingLevel"=w614:dbl)
            n227 = Unbundle By Name(w617) -> ("AIs"=w618:refnum<class "AI.lvclass">[])
            n228 = Index Array(array=w618, index=w619) -> (element=w620:refnum<class "AI.lvclass">)
            n229 = call "Get_Values.vi"("reference in"=w620) -> ("Data"=w621:T9)  [unwired: 14 in]
            n230 = Add(x=w615, y=w614) -> (x+y=w612:dbl)
            n231 = Unbundle By Name(w621) -> ("Stat Data.scl mean 1Hz"=w613:dbl)
            n232 = Greater?(x=w613, y=w612) -> (0:w604:bool)
            n233 = Select(t=Step_Name."IDLE" ("stepName"), s=w604, f=w610) -> (s? t:f=w609:T1)
            n234 = case shown="True" w604 {
              tunnel: w608 -> [w624 w629]
              tunnel: [w624 w628] -> w607
              tunnel: w606 -> [w625 w627]
              tunnel: [w625 w626] -> w605
              frame False {
              }
              frame True {
                n235 = for {
                  tunnel: T3[] [{"Active"=FALSE, "MotorN"=enum."M12"}, {"Active"=FALSE, "MotorN"=enum."M21"}, {"Active"=FALSE, "MotorN"=enum."M24"}] ("Array") -> [w633] mode=indexing
                  shift-right: [w632] -> w628
                  shift-left: w629 -> [w635]
                  shift-right: [w631] -> w626
                  shift-left: w627 -> [w634]
                  n236 = call "Activate Motor.vi"("reference in"=w635, "Active Motor"=w633, "error in (no error)"=w634) -> ("reference out"=w632:refnum<class "PM_Group.lvclass">, "error out"=w631:errorcluster)  [unwired: 11 in]
                }
              }
            }
          }
          frame "Low Pressure" {
            w651 = T8 0 items=["AI 0 Cooling Station Level", "AI 1 Cooling Station Temp", "AI 2 Oil Supply Level", "AI 3 Oil Supply Temp", "AI 4 ", "AI 5 Pressure Haskel", "AI 6 Pressure DUT", "AI 7 Pressure Chamber", "AI 8 Pressure Air inlet", "AI 9 Pressure Air outlet", "AI 10 Pressure Messure Line"] ("AI index")
            n237 = Unbundle By Name(w648) -> ("Filling Delta Level [%]"=w647:dbl, "BeginFilingLevel"=w646:dbl)
            n238 = Unbundle By Name(w649) -> ("AIs"=w650:refnum<class "AI.lvclass">[])
            n239 = Index Array(array=w650, index=w651) -> (element=w652:refnum<class "AI.lvclass">)
            n240 = call "Get_Values.vi"("reference in"=w652) -> ("Data"=w653:T9)  [unwired: 14 in]
            n241 = Add(x=w647, y=w646) -> (x+y=w644:dbl)
            n242 = Unbundle By Name(w653) -> ("Stat Data.scl mean 1Hz"=w645:dbl)
            n243 = Greater?(x=w645, y=w644) -> (0:w636:bool)
            n244 = Select(t=Step_Name."IDLE" ("stepName"), s=w636, f=w642) -> (s? t:f=w641:T1)
            n245 = case shown="True" w636 {
              tunnel: w640 -> [w656 w661]
              tunnel: [w656 w660] -> w639
              tunnel: w638 -> [w657 w659]
              tunnel: [w657 w658] -> w637
              frame False {
              }
              frame True {
                n246 = for {
                  tunnel: T3[] [{"Active"=FALSE, "MotorN"=enum."M12"}, {"Active"=FALSE, "MotorN"=enum."M21"}, {"Active"=FALSE, "MotorN"=enum."M24"}] ("Array") -> [w665] mode=indexing
                  shift-right: [w664] -> w660
                  shift-left: w661 -> [w667]
                  shift-right: [w663] -> w658
                  shift-left: w659 -> [w666]
                  n247 = call "Activate Motor.vi"("reference in"=w667, "Active Motor"=w665, "error in (no error)"=w666) -> ("reference out"=w664:refnum<class "PM_Group.lvclass">, "error out"=w663:errorcluster)  [unwired: 11 in]
                }
              }
            }
          }
          frame "Hi Pressure" {
            w676 = T7 9 items=["DO 0 [KP1] [M12]", "DO 1 [ON KP2] [M21]", "DO 2 [ON KP3] [M24]", "DO 3 [WATER Y18.1 [DO3]]", "DO 4 [WATER Y18.2 [DO4]]", "DO 5 [KP6 Y29.1 33.7]", "DO 6 [KP7 Y29.2 33.8]", "DO 7 [KP8 Y29.3 33.9]", "DO 8 [KP9 Y29.4  33.12]", "DO 9 [KP10 Y29.5 33.1]", "DO 10 [KP11 Y29.6 33.2]", "DO 11 [KP12 Y29.7  33.13]", "DO 12 [KP13 Y29.8  33.11]", "DO 13 [KP14 Y29.9 33.10]", "DO 14 [KP15 Y29.10  33.6]", "DO 15 [KP16 Y29.11  33.5]", "DO 16 [KP17 Y29.12  33.4]", "DO 17 [KP18 Y29.13 33.3]", "DO 18 [AIR KP19]", "DO 19 [STEP DRIVE EN KP20]", "DO 20 [KP21 Y44.1 OPEN]", "DO 21 [ KP22 Y44.1 CLOSE]", "DO 22 [ KP23 Y44.2 OPEN]", "DO 23", "DO 24 [STEP DRIVE 1]", "DO 25 [STEP DRIVE 2]"] ("DO index")
            n248 = call-dynamic "Read DO.vi"("FPGA API in"=w679, "error in (no error)"=w678) -> ("FPGA API out"=w670:refnum<class "FPGA API.lvclass">, "Ds"=w677:bool[], "error out"=w673:errorcluster)  [unwired: 11 in]
            n249 = Index Array(array=w677, index=w676) -> (element=w668:bool)
            n250 = Select(t=Step_Name."IDLE", s=w668, f=w675) -> (s? t:f=w672:T1)
            n251 = case shown="True" w668 {
              tunnel: w673 -> [w683 w686]
              tunnel: w671 -> [_ _]
              tunnel: w670 -> [_ w687]
              tunnel: [w683 w684] -> w669
              frame False {
              }
              frame True {
                n252 = call-dynamic "Enable Close Inlet.vi"("FPGA API in"=w687, "error in (no error)"=w686, "Direction"=Direction."None") -> ("error out"=w684:errorcluster)  [unwired: 11 in, 1 out]
              }
            }
          }
          frame "Abrupt Pressure Release" {
          }
          frame "Measuring Leakage Sensor 41.3" {
          }
          frame "Smooth Pressure Release" {
          }
          frame "Stop Pump" {
            n253 = for {
              tunnel: T3[] [{"Active"=FALSE, "MotorN"=enum."M12"}, {"Active"=FALSE, "MotorN"=enum."M21"}, {"Active"=FALSE, "MotorN"=enum."M24"}] ("Array") -> [w713] mode=indexing
              shift-right: [w712] -> w705
              shift-left: w707 -> [w715]
              shift-right: [w711] -> w704
              shift-left: w706 -> [w714]
              n254 = call "Activate Motor.vi"("reference in"=w715, "Active Motor"=w713, "error in (no error)"=w714) -> ("reference out"=w712:refnum<class "PM_Group.lvclass">, "error out"=w711:errorcluster)  [unwired: 11 in]
            }
          }
          frame "IDLE" {
          }
          frame "Measuring Leakage Burette 42" {
          }
          frame "Smooth Pressure Release" {
            n255 = disable-structure shown="Enabled" {
              disable-tunnel: w733 -> [w762 w794]
              disable-tunnel: w732 -> [w761 w786]
              disable-tunnel: w731 -> [w759 w782]
              disable-tunnel: [w755 w783] -> w730
              disable-tunnel: [w754 w784] -> w729
              disable-tunnel: w728 -> [w753 _]
              disable-tunnel: w727 -> [w740 w799]
              disable-tunnel: w726 -> [_ w788]
              frame Disabled {
                w750 = T7 24 items=["DO 0 [KP1] [M12]", "DO 1 [ON KP2] [M21]", "DO 2 [ON KP3] [M24]", "DO 3 [WATER Y18.1 [DO3]]", "DO 4 [WATER Y18.2 [DO4]]", "DO 5 [KP6 Y29.1 33.7]", "DO 6 [KP7 Y29.2 33.8]", "DO 7 [KP8 Y29.3 33.9]", "DO 8 [KP9 Y29.4  33.12]", "DO 9 [KP10 Y29.5 33.1]", "DO 10 [KP11 Y29.6 33.2]", "DO 11 [KP12 Y29.7  33.13]", "DO 12 [KP13 Y29.8  33.11]", "DO 13 [KP14 Y29.9 33.10]", "DO 14 [KP15 Y29.10  33.6]", "DO 15 [KP16 Y29.11  33.5]", "DO 16 [KP17 Y29.12  33.4]", "DO 17 [KP18 Y29.13 33.3]", "DO 18 [AIR KP19]", "DO 19 [STEP DRIVE EN KP20]", "DO 20 [KP21 Y44.1 OPEN]", "DO 21 [ KP22 Y44.1 CLOSE]", "DO 22 [ KP23 Y44.2 OPEN]", "DO 23", "DO 24 [STEP DRIVE 1]", "DO 25 [STEP DRIVE 2]"] ("DO index")
                w760 = T7 17 items=["DO 0 [KP1] [M12]", "DO 1 [ON KP2] [M21]", "DO 2 [ON KP3] [M24]", "DO 3 [WATER Y18.1 [DO3]]", "DO 4 [WATER Y18.2 [DO4]]", "DO 5 [KP6 Y29.1 33.7]", "DO 6 [KP7 Y29.2 33.8]", "DO 7 [KP8 Y29.3 33.9]", "DO 8 [KP9 Y29.4  33.12]", "DO 9 [KP10 Y29.5 33.1]", "DO 10 [KP11 Y29.6 33.2]", "DO 11 [KP12 Y29.7  33.13]", "DO 12 [KP13 Y29.8  33.11]", "DO 13 [KP14 Y29.9 33.10]", "DO 14 [KP15 Y29.10  33.6]", "DO 15 [KP16 Y29.11  33.5]", "DO 16 [KP17 Y29.12  33.4]", "DO 17 [KP18 Y29.13 33.3]", "DO 18 [AIR KP19]", "DO 19 [STEP DRIVE EN KP20]", "DO 20 [KP21 Y44.1 OPEN]", "DO 21 [ KP22 Y44.1 CLOSE]", "DO 22 [ KP23 Y44.2 OPEN]", "DO 23", "DO 24 [STEP DRIVE 1]", "DO 25 [STEP DRIVE 2]"] ("DO index")
                n256 = Unbundle By Name(w753) -> ("LinealFitting DUT"=w739:refnum<class "LinealFitting.lvclass">, "dP_dT [MPa_s]"=w747:dbl)
                n257 = call-dynamic "Read DO.vi"("FPGA API in"=w762, "error in (no error)"=w761) -> ("FPGA API out"=w752:refnum<class "FPGA API.lvclass">, "Ds"=w751:bool[], "error out"=w757:errorcluster)  [unwired: 11 in]
                n258 = call "Read Data.vi"("NeedleValve in"=w740) -> ("data value"=w745:T12)  [unwired: 10 in]
                n259 = Unbundle By Name(w745) -> ("StateValveModbus"=w744:T6)
                n260 = Index Array(array=w751, index=w750) -> (element=w748:bool)
                n261 = Index Array(array=w751, index=w760) -> (element=w756:bool)
                n262 = call "Read data.vi"("LinealFitting in"=w739) -> ("slope"=w738:dbl)  [unwired: 9 in, 1 out]
                n263 = Negate(x=w738) -> (-x=w737:dbl)
                n264 = Not Equal?(x=w744, y=Needle_Valve_State."OPENING") -> (x != y?=w742:bool)
                n265 = Greater?(x=w737, y=w747) -> (0:w741:bool)
                n266 = Select(t=Step_Name."IDLE", s=w756, f=w759) -> (s? t:f=w755:T1)
                n267 = Compound Arithmetic op=AND(invert w748, w741) -> (w749:bool)
                n268 = Compound Arithmetic op=AND(invert w748, invert w741, w742) -> (w746:bool)
                n269 = case shown="True" w746 {
                  tunnel: w740 -> [_ w763]
                  frame False {
                  }
                  frame True {
                    n270 = call "GetMessageInterface.vi"("Device in"=w763) -> ("MessageInterface"=w765:refnum<class "MessageInterface.lvclass">)  [unwired: 10 in]
                    n271 = call-dynamic "SendLocalMsg.vi"("reference in"=w765, "name"="OPEN") -> ()  [unwired: 11 in, 3 out]
                  }
                }
                n272 = case shown="True" w756 {
                  tunnel: w757 -> [w770 w778]
                  tunnel: w752 -> [_ w781]
                  tunnel: [w770 w771] -> w754
                  frame False {
                  }
                  frame True {
                    w774 = T7 24 items=["DO 0 [KP1] [M12]", "DO 1 [ON KP2] [M21]", "DO 2 [ON KP3] [M24]", "DO 3 [WATER Y18.1 [DO3]]", "DO 4 [WATER Y18.2 [DO4]]", "DO 5 [KP6 Y29.1 33.7]", "DO 6 [KP7 Y29.2 33.8]", "DO 7 [KP8 Y29.3 33.9]", "DO 8 [KP9 Y29.4  33.12]", "DO 9 [KP10 Y29.5 33.1]", "DO 10 [KP11 Y29.6 33.2]", "DO 11 [KP12 Y29.7  33.13]", "DO 12 [KP13 Y29.8  33.11]", "DO 13 [KP14 Y29.9 33.10]", "DO 14 [KP15 Y29.10  33.6]", "DO 15 [KP16 Y29.11  33.5]", "DO 16 [KP17 Y29.12  33.4]", "DO 17 [KP18 Y29.13 33.3]", "DO 18 [AIR KP19]", "DO 19 [STEP DRIVE EN KP20]", "DO 20 [KP21 Y44.1 OPEN]", "DO 21 [ KP22 Y44.1 CLOSE]", "DO 22 [ KP23 Y44.2 OPEN]", "DO 23", "DO 24 [STEP DRIVE 1]", "DO 25 [STEP DRIVE 2]"] ("#DO")
                    w779 = Direction."None" ("Direction")
                    n273 = call-dynamic "Enable Close Outlet.vi"("FPGA API in"=w781, "error in (no error)"=w778, "Direction"=w779) -> ("FPGA API out"=w780:refnum<class "FPGA API.lvclass">, "error out"=w777:errorcluster)  [unwired: 11 in]
                    n274 = call-dynamic "Enable Stop Step.vi"("FPGA API in"=w780, "error in (no error)"=w777, "Direction"=w779) -> ("FPGA API out"=w772:refnum<class "FPGA API.lvclass">, "error out"=w773:errorcluster)  [unwired: 11 in]
                    n275 = call-dynamic "Write Do.vi"("FPGA API in"=w772, "#DO"=w774, "value"=TRUE, "Time uSec"=u32 500000, "error in (no error)"=w773) -> ("error out"=w771:errorcluster)  [unwired: 9 in, 1 out]
                  }
                }
                n276 = case shown="True" w749 {
                  tunnel: w752 -> [_ w766]
                  frame False {
                  }
                  frame True {
                    w769 = T7 24 items=["DO 0 [KP1] [M12]", "DO 1 [ON KP2] [M21]", "DO 2 [ON KP3] [M24]", "DO 3 [WATER Y18.1 [DO3]]", "DO 4 [WATER Y18.2 [DO4]]", "DO 5 [KP6 Y29.1 33.7]", "DO 6 [KP7 Y29.2 33.8]", "DO 7 [KP8 Y29.3 33.9]", "DO 8 [KP9 Y29.4  33.12]", "DO 9 [KP10 Y29.5 33.1]", "DO 10 [KP11 Y29.6 33.2]", "DO 11 [KP12 Y29.7  33.13]", "DO 12 [KP13 Y29.8  33.11]", "DO 13 [KP14 Y29.9 33.10]", "DO 14 [KP15 Y29.10  33.6]", "DO 15 [KP16 Y29.11  33.5]", "DO 16 [KP17 Y29.12  33.4]", "DO 17 [KP18 Y29.13 33.3]", "DO 18 [AIR KP19]", "DO 19 [STEP DRIVE EN KP20]", "DO 20 [KP21 Y44.1 OPEN]", "DO 21 [ KP22 Y44.1 CLOSE]", "DO 22 [ KP23 Y44.2 OPEN]", "DO 23", "DO 24 [STEP DRIVE 1]", "DO 25 [STEP DRIVE 2]"] ("#DO")
                    n277 = call-dynamic "Write Do.vi"("FPGA API in"=w766, "#DO"=w769, "value"=TRUE, "Time uSec"=u32 1000000) -> ()  [unwired: 10 in, 2 out]
                  }
                }
              }
              frame Enabled {
                n278 = call "Read Data.vi"("NeedleValve in"=w799) -> ("data value"=w798:T12)  [unwired: 10 in]
                n279 = Unbundle By Name(w788) -> ("P MB DUT"=w791:refnum<class "AI.lvclass">)
                n280 = Unbundle By Name(w798) -> ("Angele"=w797:dbl)
                n281 = call "Get_Values.vi"("reference in"=w791) -> ("Data"=w790:T9)  [unwired: 14 in]
                n282 = Greater?(x=w797, y=40.0) -> (0:w795:bool)
                n283 = Unbundle By Name(w788) -> ("Pressure SP"=w787:dbl)
                n284 = Unbundle By Name(w790) -> ("Stat Data.scl mean"=w789:dbl)
                n285 = case shown="True" w795 {
                  tunnel: w794 -> [w808 w812]
                  tunnel: [w808 w811] -> w793
                  tunnel: [w807 w810] -> w792
                  tunnel: w786 -> [w807 w809]
                  frame False {
                  }
                  frame True {
                    n286 = call-dynamic "Enable Stop Step.vi"("FPGA API in"=w812, "error in (no error)"=w809, "Direction"=Direction."DUT") -> ("FPGA API out"=w811:refnum<class "FPGA API.lvclass">, "error out"=w810:errorcluster)  [unwired: 11 in]
                  }
                }
                n287 = Less Or Equal?(x=w789, y=w787) -> (x <= y?=w785:bool)
                n288 = case shown="True" w785 {
                  tunnel: w793 -> [_ w806]
                  tunnel: w792 -> [w801 w805]
                  tunnel: [w801 w803] -> w784
                  tunnel: [w800 Step_Name."IDLE" ("STEP")] -> w783
                  tunnel: w782 -> [w800 _]
                  frame False {
                  }
                  frame True {
                    w804 = T7[] [] items=["DO 0 [KP1] [M12]", "DO 1 [ON KP2] [M21]", "DO 2 [ON KP3] [M24]", "DO 3 [WATER Y18.1 [DO3]]", "DO 4 [WATER Y18.2 [DO4]]", "DO 5 [KP6 Y29.1 33.7]", "DO 6 [KP7 Y29.2 33.8]", "DO 7 [KP8 Y29.3 33.9]", "DO 8 [KP9 Y29.4  33.12]", "DO 9 [KP10 Y29.5 33.1]", "DO 10 [KP11 Y29.6 33.2]", "DO 11 [KP12 Y29.7  33.13]", "DO 12 [KP13 Y29.8  33.11]", "DO 13 [KP14 Y29.9 33.10]", "DO 14 [KP15 Y29.10  33.6]", "DO 15 [KP16 Y29.11  33.5]", "DO 16 [KP17 Y29.12  33.4]", "DO 17 [KP18 Y29.13 33.3]", "DO 18 [AIR KP19]", "DO 19 [STEP DRIVE EN KP20]", "DO 20 [KP21 Y44.1 OPEN]", "DO 21 [ KP22 Y44.1 CLOSE]", "DO 22 [ KP23 Y44.2 OPEN]", "DO 23", "DO 24 [STEP DRIVE 1]", "DO 25 [STEP DRIVE 2]"] ("#DO")
                    n289 = call "DoValve.vi"("reference in"=w806, 5:w804, "error in (no error)"=w805) -> ("error out"=w803:errorcluster)  [unwired: 11 in, 1 out]
                  }
                }
              }
            }
          }
          frame "Alarm" {
            n290 = call "Config Setpoints.vi"("reference in"=w826) -> ()  [unwired: 14 in, 1 out]
            n291 = Unbundle By Name(w822) -> ("AIs"=w823:refnum<class "AI.lvclass">[], "Pressure SP"=w818:dbl)
            n292 = Index Array(array=w823, index=6) -> (element=w821:refnum<class "AI.lvclass">)
            n293 = call "Get_Values.vi"("reference in"=w821) -> ("Data"=w820:T9)  [unwired: 14 in]
            n294 = Unbundle By Name(w820) -> ("Stat Data.scl mean 1Hz"=w819:dbl)
            n295 = Greater?(x=w819, y=w818) -> (0:w817:bool)
            n296 = case shown="False" w817 {
              tunnel: w816 -> [w836 w844]
              tunnel: [w832 w840] -> w815
              tunnel: w814 -> [w830 w838]
              frame True {
                w837 = T7[] [17, 6] items=["DO 0 [KP1] [M12]", "DO 1 [ON KP2] [M21]", "DO 2 [ON KP3] [M24]", "DO 3 [WATER Y18.1 [DO3]]", "DO 4 [WATER Y18.2 [DO4]]", "DO 5 [KP6 Y29.1 33.7]", "DO 6 [KP7 Y29.2 33.8]", "DO 7 [KP8 Y29.3 33.9]", "DO 8 [KP9 Y29.4  33.12]", "DO 9 [KP10 Y29.5 33.1]", "DO 10 [KP11 Y29.6 33.2]", "DO 11 [KP12 Y29.7  33.13]", "DO 12 [KP13 Y29.8  33.11]", "DO 13 [KP14 Y29.9 33.10]", "DO 14 [KP15 Y29.10  33.6]", "DO 15 [KP16 Y29.11  33.5]", "DO 16 [KP17 Y29.12  33.4]", "DO 17 [KP18 Y29.13 33.3]", "DO 18 [AIR KP19]", "DO 19 [STEP DRIVE EN KP20]", "DO 20 [KP21 Y44.1 OPEN]", "DO 21 [ KP22 Y44.1 CLOSE]", "DO 22 [ KP23 Y44.2 OPEN]", "DO 23", "DO 24 [STEP DRIVE 1]", "DO 25 [STEP DRIVE 2]"] ("#DO")
                n297 = call-dynamic "Enable Close Outlet.vi"("FPGA API in"=w836, "error in (no error)"=w830, "Direction"=Direction."DUT") -> ("FPGA API out"=w833:refnum<class "FPGA API.lvclass">, "error out"=w834:errorcluster)  [unwired: 11 in]
                n298 = call "DoValve.vi"("reference in"=w833, 5:w837, 7:u32 0 ("Time uSec"), "error in (no error)"=w834) -> ("error out"=w832:errorcluster)  [unwired: 10 in, 1 out]
              }
              frame False {
                w845 = T7[] [] items=["DO 0 [KP1] [M12]", "DO 1 [ON KP2] [M21]", "DO 2 [ON KP3] [M24]", "DO 3 [WATER Y18.1 [DO3]]", "DO 4 [WATER Y18.2 [DO4]]", "DO 5 [KP6 Y29.1 33.7]", "DO 6 [KP7 Y29.2 33.8]", "DO 7 [KP8 Y29.3 33.9]", "DO 8 [KP9 Y29.4  33.12]", "DO 9 [KP10 Y29.5 33.1]", "DO 10 [KP11 Y29.6 33.2]", "DO 11 [KP12 Y29.7  33.13]", "DO 12 [KP13 Y29.8  33.11]", "DO 13 [KP14 Y29.9 33.10]", "DO 14 [KP15 Y29.10  33.6]", "DO 15 [KP16 Y29.11  33.5]", "DO 16 [KP17 Y29.12  33.4]", "DO 17 [KP18 Y29.13 33.3]", "DO 18 [AIR KP19]", "DO 19 [STEP DRIVE EN KP20]", "DO 20 [KP21 Y44.1 OPEN]", "DO 21 [ KP22 Y44.1 CLOSE]", "DO 22 [ KP23 Y44.2 OPEN]", "DO 23", "DO 24 [STEP DRIVE 1]", "DO 25 [STEP DRIVE 2]"] ("#DO")
                n299 = call-dynamic "Enable Close Outlet.vi"("FPGA API in"=w844, "error in (no error)"=w838, "Direction"=Direction."DUT") -> ("FPGA API out"=w841:refnum<class "FPGA API.lvclass">, "error out"=w842:errorcluster)  [unwired: 11 in]
                n300 = call "DoValve.vi"("reference in"=w841, 5:w845, 7:u32 0 ("Time uSec"), "error in (no error)"=w842) -> ("error out"=w840:errorcluster)  [unwired: 10 in, 1 out]
              }
            }
          }
          frame "Measuring Leakage Sensor 41.3" {
            w853 = T7 10 items=["DO 0 [KP1] [M12]", "DO 1 [ON KP2] [M21]", "DO 2 [ON KP3] [M24]", "DO 3 [WATER Y18.1 [DO3]]", "DO 4 [WATER Y18.2 [DO4]]", "DO 5 [KP6 Y29.1 33.7]", "DO 6 [KP7 Y29.2 33.8]", "DO 7 [KP8 Y29.3 33.9]", "DO 8 [KP9 Y29.4  33.12]", "DO 9 [KP10 Y29.5 33.1]", "DO 10 [KP11 Y29.6 33.2]", "DO 11 [KP12 Y29.7  33.13]", "DO 12 [KP13 Y29.8  33.11]", "DO 13 [KP14 Y29.9 33.10]", "DO 14 [KP15 Y29.10  33.6]", "DO 15 [KP16 Y29.11  33.5]", "DO 16 [KP17 Y29.12  33.4]", "DO 17 [KP18 Y29.13 33.3]", "DO 18 [AIR KP19]", "DO 19 [STEP DRIVE EN KP20]", "DO 20 [KP21 Y44.1 OPEN]", "DO 21 [ KP22 Y44.1 CLOSE]", "DO 22 [ KP23 Y44.2 OPEN]", "DO 23", "DO 24 [STEP DRIVE 1]", "DO 25 [STEP DRIVE 2]"] ("DO index")
            n301 = call-dynamic "Read DO.vi"("FPGA API in"=w856, "error in (no error)"=w855) -> ("FPGA API out"=w847:refnum<class "FPGA API.lvclass">, "Ds"=w854:bool[], "error out"=w850:errorcluster)  [unwired: 11 in]
            n302 = Index Array(array=w854, index=w853) -> (element=w849:bool)
            n303 = Select(t=Step_Name."IDLE", s=w849, f=w852) -> (s? t:f=w848:T1)
            n304 = case shown="True" w849 {
              tunnel: w850 -> [w860 w863]
              tunnel: w847 -> [_ w864]
              tunnel: [w860 w861] -> w846
              frame False {
              }
              frame True {
                n305 = call-dynamic "Enable Close Inlet.vi"("FPGA API in"=w864, "error in (no error)"=w863, "Direction"=Direction."None") -> ("error out"=w861:errorcluster)  [unwired: 11 in, 1 out]
              }
            }
          }
          frame "Measuring Leakage Burette 42" {
          }
          frame "Alarm" {
            w870 = T7 24 items=["DO 0 [KP1] [M12]", "DO 1 [ON KP2] [M21]", "DO 2 [ON KP3] [M24]", "DO 3 [WATER Y18.1 [DO3]]", "DO 4 [WATER Y18.2 [DO4]]", "DO 5 [KP6 Y29.1 33.7]", "DO 6 [KP7 Y29.2 33.8]", "DO 7 [KP8 Y29.3 33.9]", "DO 8 [KP9 Y29.4  33.12]", "DO 9 [KP10 Y29.5 33.1]", "DO 10 [KP11 Y29.6 33.2]", "DO 11 [KP12 Y29.7  33.13]", "DO 12 [KP13 Y29.8  33.11]", "DO 13 [KP14 Y29.9 33.10]", "DO 14 [KP15 Y29.10  33.6]", "DO 15 [KP16 Y29.11  33.5]", "DO 16 [KP17 Y29.12  33.4]", "DO 17 [KP18 Y29.13 33.3]", "DO 18 [AIR KP19]", "DO 19 [STEP DRIVE EN KP20]", "DO 20 [KP21 Y44.1 OPEN]", "DO 21 [ KP22 Y44.1 CLOSE]", "DO 22 [ KP23 Y44.2 OPEN]", "DO 23", "DO 24 [STEP DRIVE 1]", "DO 25 [STEP DRIVE 2]"] ("DO index")
            w879 = T7 16 items=["DO 0 [KP1] [M12]", "DO 1 [ON KP2] [M21]", "DO 2 [ON KP3] [M24]", "DO 3 [WATER Y18.1 [DO3]]", "DO 4 [WATER Y18.2 [DO4]]", "DO 5 [KP6 Y29.1 33.7]", "DO 6 [KP7 Y29.2 33.8]", "DO 7 [KP8 Y29.3 33.9]", "DO 8 [KP9 Y29.4  33.12]", "DO 9 [KP10 Y29.5 33.1]", "DO 10 [KP11 Y29.6 33.2]", "DO 11 [KP12 Y29.7  33.13]", "DO 12 [KP13 Y29.8  33.11]", "DO 13 [KP14 Y29.9 33.10]", "DO 14 [KP15 Y29.10  33.6]", "DO 15 [KP16 Y29.11  33.5]", "DO 16 [KP17 Y29.12  33.4]", "DO 17 [KP18 Y29.13 33.3]", "DO 18 [AIR KP19]", "DO 19 [STEP DRIVE EN KP20]", "DO 20 [KP21 Y44.1 OPEN]", "DO 21 [ KP22 Y44.1 CLOSE]", "DO 22 [ KP23 Y44.2 OPEN]", "DO 23", "DO 24 [STEP DRIVE 1]", "DO 25 [STEP DRIVE 2]"] ("DO index")
            n306 = call-dynamic "Read DO.vi"("FPGA API in"=w882, "error in (no error)"=w881) -> ("FPGA API out"=w872:refnum<class "FPGA API.lvclass">, "Ds"=w880:bool[], "error out"=w876:errorcluster)  [unwired: 11 in]
            n307 = Index Array(array=w880, index #1=w879, index #2=w870) -> (element #1=w875:bool)  [unwired: 1 out]
            n308 = Select(t=Step_Name."IDLE", s=w875, f=w878) -> (s? t:f=w874:T1)
            n309 = case shown="True" w875 {
              tunnel: w876 -> [w886 w889]
              tunnel: w873 -> [_ _]
              tunnel: w872 -> [_ w892]
              tunnel: [w886 w887] -> w871
              frame False {
              }
              frame True {
                w890 = Direction."None" ("Direction")
                n310 = call-dynamic "Enable Close Outlet.vi"("FPGA API in"=w892, "error in (no error)"=w889, "Direction"=w890) -> ("FPGA API out"=w891:refnum<class "FPGA API.lvclass">, "error out"=w888:errorcluster)  [unwired: 11 in]
                n311 = call-dynamic "Enable Stop Step.vi"("FPGA API in"=w891, "error in (no error)"=w888, "Direction"=w890) -> ("error out"=w887:errorcluster)  [unwired: 11 in, 1 out]
              }
            }
          }
          frame "Stop Pump" {
          }
          frame "Abrupt Pressure Release" {
            w899 = T7[] [8, 17, 10] items=["DO 0 [KP1] [M12]", "DO 1 [ON KP2] [M21]", "DO 2 [ON KP3] [M24]", "DO 3 [WATER Y18.1 [DO3]]", "DO 4 [WATER Y18.2 [DO4]]", "DO 5 [KP6 Y29.1 33.7]", "DO 6 [KP7 Y29.2 33.8]", "DO 7 [KP8 Y29.3 33.9]", "DO 8 [KP9 Y29.4  33.12]", "DO 9 [KP10 Y29.5 33.1]", "DO 10 [KP11 Y29.6 33.2]", "DO 11 [KP12 Y29.7  33.13]", "DO 12 [KP13 Y29.8  33.11]", "DO 13 [KP14 Y29.9 33.10]", "DO 14 [KP15 Y29.10  33.6]", "DO 15 [KP16 Y29.11  33.5]", "DO 16 [KP17 Y29.12  33.4]", "DO 17 [KP18 Y29.13 33.3]", "DO 18 [AIR KP19]", "DO 19 [STEP DRIVE EN KP20]", "DO 20 [KP21 Y44.1 OPEN]", "DO 21 [ KP22 Y44.1 CLOSE]", "DO 22 [ KP23 Y44.2 OPEN]", "DO 23", "DO 24 [STEP DRIVE 1]", "DO 25 [STEP DRIVE 2]"] ("#DO")
            # "Замер утечек из образца по датчику 41.3\n4.1\tконтроль показаний\n4.2\tконтроль показаний\n5.1\tконтроль показаний\n5.2\tконтроль показаний\n12\t0/1\n18.1\t0/1\n18.2\t0/1\n21\t1\n24\t0/1\n25\t1\n29.1 (33.7)\t0\n29.2 (33.8)\t0\n29.3 (33.9)\t0\n29.4 (33.12)\t1\n29.5 (33.1)\t0\n29.6 (33.2)\t1\n29.7 (33.13)\t0\n29.8 (33.11)\t0\n29.9 (33.10)\t0\n29.10 (33.6)\t0\n29.11 (33.5)\t0\n29.12 (33.4)\t0\n29.13 (33.3) \t1\n30\t0…10 В\n35.1\t60%\n35.2\t0\n36.1\tконтроль показаний\n36.2\tконтроль показаний\n38.1\tконтроль показаний\n38.2\tконтроль показаний\n38.3\tобратная связь\n41.3\tконтроль показаний\n44.1\t0\n44.2\t0\n46\t0…1,5 В"
            # "OPEN"
            # "CLOSE"
            # "STOP"
            n312 = Unbundle By Name(w928) -> ("Pressure SP"=w906:dbl)
            n313 = call "Config Setpoints.vi"("reference in"=w902, "error in (no error)"=w901) -> ("error out"=w900:errorcluster)  [unwired: 13 in]
            n314 = call "Pressure to voltage.vi"("Pressure SP"=w906) -> ()  [unwired: 14 in, 1 out]
            n315 = call "DoValve.vi"("reference in"=w931, 5:w899, "error in (no error)"=w900) -> ("reference out"=w935:refnum<class "FPGA API.lvclass">, "error out"=w934:errorcluster)  [unwired: 11 in]
            n316 = call-dynamic "SetHasckelAO.vi"("FPGA API in"=w935, "Haskel in"=0.0, "error in (no error)"=w934) -> ("FPGA API out"=w933:refnum<class "FPGA API.lvclass">, "error out"=w932:errorcluster)  [unwired: 11 in]
            n317 = call-dynamic "SetPropValve.vi"("FPGA API in"=w933, "AO 1"=0.0, "error in (no error)"=w932) -> ("FPGA API out"=w918:refnum<class "FPGA API.lvclass">, "error out"=w917:errorcluster)  [unwired: 11 in]
            n318 = call-dynamic "Enable Close Inlet.vi"("FPGA API in"=w918, "error in (no error)"=w917, "Direction"=Direction."None") -> ("FPGA API out"=w915:refnum<class "FPGA API.lvclass">, "error out"=w914:errorcluster)  [unwired: 11 in]
            n319 = call-dynamic "Enable Close Outlet.vi"("FPGA API in"=w915, "error in (no error)"=w914, "Direction"=Direction."Chamber") -> ("FPGA API out"=w912:refnum<class "FPGA API.lvclass">, "error out"=w911:errorcluster)  [unwired: 11 in]
            n320 = call-dynamic "Enable Stop Step.vi"("FPGA API in"=w912, "error in (no error)"=w911, "Direction"=Direction."Chamber") -> ("error out"=w910:errorcluster)  [unwired: 11 in, 1 out]
            n321 = disable-structure shown="Disabled" {
              disable-tunnel: w921 -> [w939 _]
              disable-tunnel: [w938 _] -> w920
              frame Disabled {
                n322 = call "GetMessageInterface.vi"("Device in"=w939) -> ("MessageInterface"=w937:refnum<class "MessageInterface.lvclass">)  [unwired: 10 in]
                n323 = call-dynamic "SendLocalMsg.vi"("reference in"=w937, "name"="") -> ("error out"=w938:errorcluster)  [unwired: 11 in, 2 out]
              }
              frame Enabled {
              }
            }
            n324 = call "GetMessageInterface.vi"("Device in"=w919) -> ("MessageInterface"=w904:refnum<class "MessageInterface.lvclass">)  [unwired: 10 in]
            n325 = call "Close.vi"("Pump_1AI_1DO_2DI in"=w930) -> ("error out"=w922:errorcluster, "Pump_1AI_1DO_2DI out"=w927:refnum<class "Valve_2DO_2DI.lvclass">)  [unwired: 9 in]
            n326 = call "Close.vi"("Pump_1AI_1DO_2DI in"=w926) -> ("error out"=w923:errorcluster, "Pump_1AI_1DO_2DI out"=w925:refnum<class "Valve_2DO_2DI.lvclass">)  [unwired: 9 in]
            n327 = call-dynamic "SendLocalMsg.vi"("reference in"=w904, "name"="OPEN") -> ("error out"=w908:errorcluster)  [unwired: 11 in, 2 out]
            n328 = Merge Errors(w910, w922, w923, w920, w908) -> (w924:errorcluster)
          }
          frame "Low Pressure" {
            w942 = T8 6 items=["AI 0 Cooling Station Level", "AI 1 Cooling Station Temp", "AI 2 Oil Supply Level", "AI 3 Oil Supply Temp", "AI 4 ", "AI 5 Pressure Haskel", "AI 6 Pressure DUT", "AI 7 Pressure Chamber", "AI 8 Pressure Air inlet", "AI 9 Pressure Air outlet", "AI 10 Pressure Messure Line"] ("AI index")
            n329 = call "Set Low Press.vi"("reference in"=w941, "AI index"=w942, "error in (no error)"=w943) -> ("error out"=w944:errorcluster)  [unwired: 12 in]
          }
          frame "Filling" {
            w950 = T8 7 items=["AI 0 Cooling Station Level", "AI 1 Cooling Station Temp", "AI 2 Oil Supply Level", "AI 3 Oil Supply Temp", "AI 4 ", "AI 5 Pressure Haskel", "AI 6 Pressure DUT", "AI 7 Pressure Chamber", "AI 8 Pressure Air inlet", "AI 9 Pressure Air outlet", "AI 10 Pressure Messure Line"] ("AI index")
            n330 = call "Set Low Press.vi"("reference in"=w949, "AI index"=w950, "error in (no error)"=w951) -> ("error out"=w952:errorcluster)  [unwired: 12 in]
          }
          frame "Hi Pressure" {
            w958 = T8 5 items=["AI 0 Cooling Station Level", "AI 1 Cooling Station Temp", "AI 2 Oil Supply Level", "AI 3 Oil Supply Temp", "AI 4 ", "AI 5 Pressure Haskel", "AI 6 Pressure DUT", "AI 7 Pressure Chamber", "AI 8 Pressure Air inlet", "AI 9 Pressure Air outlet", "AI 10 Pressure Messure Line"] ("AI index")
            n331 = call "Set Low Press.vi"("reference in"=w957, "AI index"=w958, "error in (no error)"=w959) -> ("error out"=w960:errorcluster)  [unwired: 12 in]
          }
        }
        n332 = in-place-cluster #2("MODE"=w586, "PM"=w592, "VLV 44.1"=w591, "VLV 44.2"=w590) -> (w582:refnum<class "Stand.lvclass">)
      }
    }
  }
  "error out" <- w7
  "Stand out" <- w8
